vi "FIFOScreenBurst.vi"() -> ()   [LabVIEW 2009]
uses:
  <vilib>/Utility/file.llb/Write To Spreadsheet File (DBL).vi
  <vilib>/Analysis/NI_AALBase.lvlib
  <vilib>/Analysis/NI_AALPro.lvlib
panel:
  in  "get background":bool
  in  "areas and ratio":cluster{dbl, dbl, dbl}
  in  "ratio histogram":dbl[](array[numeric]) format="%0.2f"
  in  "Case Constant\n(See Context Help) 2":bool=TRUE
  in  "Case Constant\n(See Context Help)":bool
  out "MCS":T1(graph)
  out "Lifetime bins":i32=32768
  out "HH":bool=TRUE
  in  "Export times":bool
  in  "Corellate!":bool
  in  "SPC Format":u16(ring)=3 items=["SPC 630 - 32 bit", "SPC 630 - 48 bit", "SPC 830 - 32 bit", "HydraHarp"]
  out "F2 output path":path
  out "channels":u8[](array[numeric])
  out "element":u32
  in  "Acceptor":u8=3
  in  "Transmitter 2":u8=7
  in  "Donor":u8=1
  in  "Transmitter 1":u8=6
  out "T 2":u32
  in  "Correlation":bool
  in  "File Number":u32(slide) max=17 scale=-1.1..17.0
  in  "MCS Export Path (ASCII-File)":path
  out "Busy":bool
  out "donor":i32
  out "T1":i32
  out "all photons":u32
  out "invalid":u32
  out "gaps":u32
  in  "file path":path=path "D:/data/setup test/sim.fifo"
  in  "binning / s":dbl=0.01 format="%.6f"
  out "Save F2":dbl[][](array[numeric]) format="%.2f"
  in  "Export MCS":bool
  in  "Tab Control":T2(tab)=enum."autcorrelation"
  in  "Export Traces":bool
  in  "Trace Export Path (ASCII-File)":path
  in  "shift (photons)":u32=1000
  out "traces":cluster{"SlideTime":dbl[], dbl[]}[](graph)
  out "traces":cluster{dbl, "binning":dbl, "MLE trace":dbl[]}[](graph)
  in  "binning type":u16(ring) items=["seconds", "photons"]
  in  "binning":dbl=0.002 format="%.6f"
  out "sum":u32
  in  "Export Coincidence":bool
  in  "Coincidence Export Path (ASCII-File)":path
  out "coincidence ratio":dbl format="%.2f"
  in  "lateral peaks":u32=6 min=2 max=10 step=2
  in  "center peak (µs)":dbl=1.0 format="%.2f"
  in  "histogram lenght (µs)":dbl=10.0 format="%.2f"
  out "coincidence histogram":T3(graph)
  in  "delay channel 1":bool=TRUE
  in  "TAC range (ns)":dbl=50.0
  in  "export path":path
  in  "export lifetime":bool
  in  "Export Decay":bool
  in  "export decay path":path
  out "lifetime (ns)":dbl[][](array[numeric]) format="%.2f"
  in  "rebinning":u16=1 min=1 max=4096 step=1
  in  "HH Binning / TAC Gain":u16=1
  out "lifetime histogram":T4(graph)
  in  "ch1 (0=sum)":i32
  in  "ch2":i32=1
  in  "ch3":i32=2
  out "selected photons ch3":u32
  out "max value":dbl
  in  "only selected region?":bool
  in  "Pfad":path
  in  "biExp fit":bool
  out "S+B (Hz)":i32
  in  "B":dbl=500.0 format="%.2f"
  in  "skip":i32
  out "F2":dbl
  in  "cross ch2":i32=1
  in  "auto/crossch1":i32
  in  "none/auto/cross":u8
  out "Autocorrelation":cluster{dbl[], "Best Fit":dbl[]}[](graph)
  in  "FCS-Export-Path":path=path "D:/0.001_2000ns_fcs.dat"
  out "diffusion-triplett-model":string="1/N*(1+(r/1-r)*exp(-x*t1))/(1+x/t2)*(1+x/(4*t2))^(-1/2)+o"
  out "Parameters 3":string[](array[string])=["o", "t1", "t2", "N", "r"]
  in  "Initial Guess Coefficient":dbl[](array[numeric])=[0.0, 0.01, 0.18, 0.03, 0.2] format="%.2e"
  out "Parameters 2":string[](array[string])=["o", "t1", "t2", "N", "r"]
  out "Best Fit Coefficient":dbl[][](array[numeric]) format="%.2e"
  in  "freeform":T5={"model"="((1/b)*(1+(a/(1-a))*exp(-x/t1))/(1+x/t2)*(1+x/(4*t2))^(-1/2))+o", "Parameters"=["o", "t1", "t2", "b", "a"], "x"="x"}
  in  "Fit-Type":u8
  out "on2":cluster{"Axis":dbl[], "Histogram":i32[]}(graph)
  out "ChannelsHist":cluster{"Axis":dbl[], "Histogram":i32[]}(graph)
  out "Avg off":dbl format="%.2f"
  out "Avg On":dbl format="%.2f"
  in  "Int-Threshold 2":sgl format="%.2f"
  in  "Int-Threshold":sgl=15.0 format="%.2f"
  out "Offs 0":cluster{"Axis":dbl[], "Histogram":i32[]}(graph)
  out "On plot1":cluster{"Axis":dbl[], "Histogram":i32[]}(graph)
  out "Int Histogram":cluster{"Axis":dbl[], "Histogram":i32[]}(graph)
  out "off":dbl[](array[numeric]) format="%.2f"
  out "on":dbl[](array[numeric]) format="%.2f"
  in  "min bin time (ns)":u32=1000
  in  "Export Correlation":bool
  out "results":T6
  out "Deviation":cluster{dbl[], "Best Fit":dbl[]}[](graph)
  out "Mean Intensity/\nbackground":dbl
  in  "automatic threshold":bool
  out "Statistik F2":dbl[](array[numeric])=[0.0, 0.06084751773049646, 1269.0, 0.47169755424752874, 11.13572770347884, 1.44, 1.0499999999999998, 0.035, 2.525] format="%.2f"
  out "Fn-Values":cluster{dbl, "Value":dbl, dbl[]}[](graph)
  in  "bin / s":dbl=0.5 format="%.6f"
  in  "Export F2":bool
  out "FRET histogram":cluster{"Axis":dbl[], "Histogram":i32[]}[](graph)
  in  "F2-Value Export Path":path=path "D:/Messungen/040901_VHA-Rh110_VHA-Atto590_AMP-PNP/name_1000mus_55bins.dat"
  out "# bursts":i32
  in  "# bins":i32=55
  out "Summe":cluster{"Axis":dbl[], "Histogram":i32[]}(graph)
  in  "% overtalk D-T2":u8
  in  "% overtalk D-A":u8
  in  "% overtalk D-T1":u8
  in  "* w0":u8
  out "mean, std.dev":dbl[](array[numeric])=[0.0, 0.0, -0.3793442467648379, 0.0] format="%.2f"
  in  "Parameters":T7={"PeakThreshold"=30, "RecognitionThs"=25, "SeparationLimit"=0.7} {"SeparationLimit" format="%.2f"}
  in  "Burst recognition":bool=TRUE
  in  "Save ASCII":bool
  in  "add previous":bool
  in  "Open":bool
  in  "Save":bool
  out "# off times":i32
  out "# on times":i32
  out "off time histogram":T8(graph)
  in  "intervals":i32=3
  out "on count histogram":T8(graph)
  out "StdDev":dbl format="%0.2f"
  out "off time (s)":dbl
  out "StdDev":dbl format="%_4f"
  out "off times (s)":dbl[](array[numeric]) format="%.4f"
  out "on counts":i32[](array[numeric])
  out "on time photons":dbl
  in  "channel":i32
  in  "start":bool
  in  "Export area histogram":bool
  in  "Clear histogram":bool
  in  "Add ratio":bool
  out "Histogram Graph":cluster{"X":dbl[], "Histogram":dbl[]}[](graph)
  out "ratio peak areas\nFRET high/FRET low":dbl
  in  "fitting?":bool
  out "ratio histogram":T8(graph)
  out "area low FRET":dbl
  out "area high FRET":dbl
  out "sum low":dbl
  out "sum high":dbl
  # "FifFo Screen Burst\nFour Channel extension\nv0.17"
  # "0: none\n1: diffusion\n2: freeform\n3: exponentiell"
  # "Donor"
  # "Transmitter1"
  # "Transmitter2"
  # "r is amplitude fraction of triplet"
  # "Acceptor"
  # "in ms"
  # "Spot"
  # "burst/s"
  # "bursts"
  # "mean burstwidth /ms"
  # "mean Int"
  # "rec. Thres"
  # "x"
  # "µ"
  # "2*s"
  # "calculates E= acceptor/(acceptor+donor) and fits two gaussian"
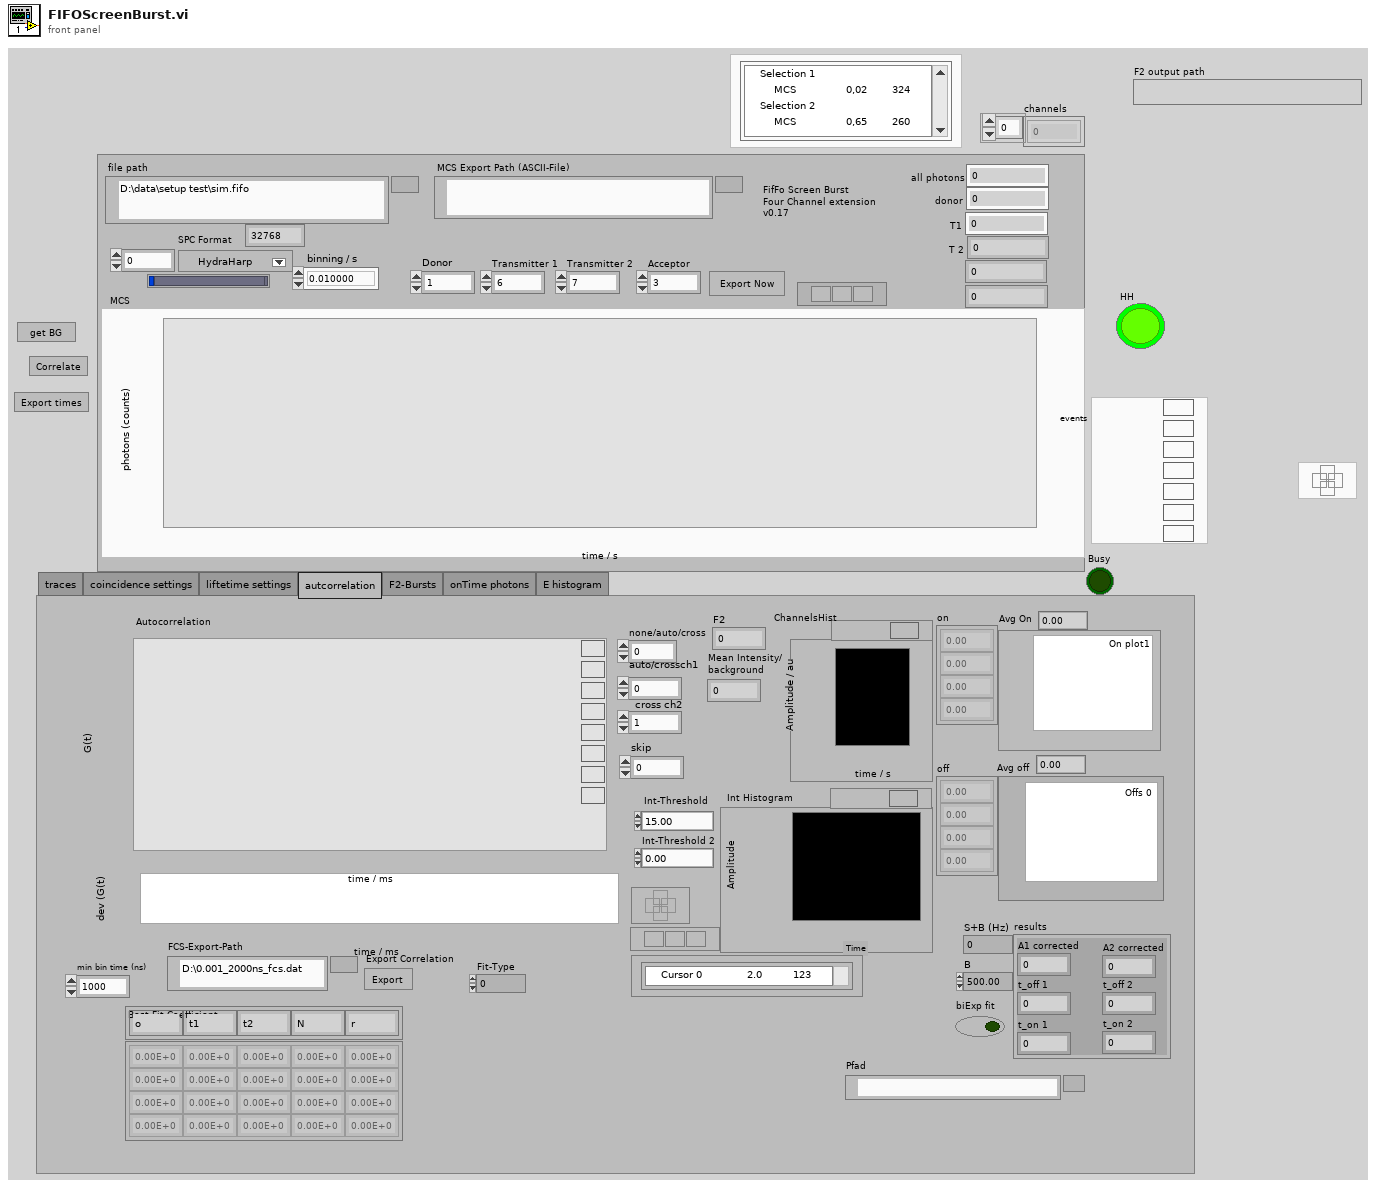
[diagram p1: front panel]
types:
  T1 = cluster{"binning (s)":dbl, "binning (s)":dbl, "Histogram: h(x)":u32[]}[]
  T2 = enum32{"traces", "coincidence settings", "liftetime settings", "autcorrelation", "F2-Bursts", "onTime photons", "E histogram"}
  T3 = cluster{"Origin (ns)":dbl, "Offset (ns)":dbl, u32[]}
  T4 = cluster{dbl, "channel width (ns)":dbl, "channel 1":u32[]}[]
  T5 = cluster{"model":string, "Parameters":string[], "x":string}
  T6 = cluster{"A1 corrected":dbl, "t_off 1":dbl, "t_on 1":dbl, "A2 corrected":dbl, "t_off 2":dbl, "t_on 2":dbl}
  T7 = cluster{"PeakThreshold":u32, "RecognitionThs":u32, "SeparationLimit":sgl}
  T8 = cluster{"X Values":dbl[], "Histogram: h(x)":i32[]}
  T9 = enum16{"open", "open or create", "create or replace", "create", "open (read only)"}
  T10 = cluster{dbl, "binning":dbl, "center peak trace":dbl[]}[]
  T11 = cluster{"SlideTime":dbl[], "SlideCenterPeak":dbl[]}[]
  T12 = cluster{"origin (ns)":dbl, "offset (ns)":dbl, "histogram":u32[]}
  T13 = typedef "Settings.ctl" = cluster{"threshold":cluster{"max":u32, "min":u32}, "RGB or false color":bool, "16bit":bool, "log/lin axis":u16, "spotsize button":bool, "Pixelsize":u16, "autoscale x":bool, "autoscale y":bool, "correlation":bool, "ADC-Resolution":i32, "F2-lifetime":cluster{"display tau":bool, "display F2":bool, "Palette Number lifetime":enum32{"Gray", "Binary", "Gradient", "Rainbow", "Temperature"}, "Palette Number F2":enum32{"Gray", "Binary", "Gradient", "Rainbow", "Temperature"}, "max tau-Value":dbl, "min tau-Value":dbl, "max F2-Value":dbl, "min F2-Value":dbl}, "TAC-Window 1":u16, "TAC-Window 2":u16, "false color palette":cluster{"1":u32, "2":u32, "3":u32, "4":u32, "5":u32, "6":u32, "7":u32, "8":u32, "8 2":u32, "8 3":u32, "8 4":u32, "8 5":u32}, "rebinning":dbl}
  T14 = cluster{"sum":u32[], "channel 0":u32[], "channel 1":u32[], "channel width (ns)":dbl}
  T15 = typedef "LVCursorListTypeDef.ctl" = cluster{"Name":string, "Color":u32, "Style":u8, "Point Style":u8, "Name Visible":bool, "Allow Drag":bool, "Cursor Mode":u32, "Plot":i32, "Index":i32, "Position":cluster{"X":dbl, "Y":dbl}, "X Scale":u32, "Y Scale":u32, "Watch Plots":i32[], "Watch All Plots":bool, "Plot Area":i32, "Label Offset":cluster{"X":dbl, "Y":dbl}}[]
  T16 = cluster{"router channels":u8[], "macro times":dbl[], "micro times":u16[], "invalid times":u32[], "gap times":u32[]}
  T17 = cluster{"Name":string, "Color":u32, "Style":u8, "Point Style":u8, "Name Visible":bool, "Allow Drag":bool, "Cursor Mode":u32, "Plot":i32, "Index":i32, "Position":cluster{"X":dbl, "Y":dbl}, "X Scale":u32, "Y Scale":u32, "Watch Plots":i32[], "Watch All Plots":bool, "Plot Area":i32, "Label Offset":cluster{"X":dbl, "Y":dbl}}
  T18 = cluster{"binning (s)":dbl, "binning (s)":dbl, "Histogram: h(x)":u32[]}
  T19 = cluster{"router channels":u8[], "macro times(50ns steps)":u32[], "micro times":u16[], "invalid times":u32[], "gap times":u32[]}
  T20 = cluster{"router channels":u8[], "macro times":u32[], "micro times":u16[], "invalid times":u32[], "gap times":u32[]}
  T21 = cluster{"binning (s)":dbl, "binning (s)":dbl, "Histogram: h(x)":i32[]}
  T22 = cluster{"offset":dbl, "binning (s)":dbl, "MCS":u32[]}
  T23 = cluster{"binning (s)":dbl, "binning (s)":dbl, "MCS":u32[]}[]
  T24 = cluster{dbl, "binning":dbl, "coincidence trace":dbl[]}
  T25 = cluster{dbl, "binning":dbl, "center peak trace":u32[]}
  T26 = cluster{dbl, "binning":dbl, "coincidence trace":dbl[]}[]
  T27 = cluster{"SlideTime":dbl[], "SlideLifetime":dbl[]}
  T28 = cluster{"SlideTime":dbl[], "SlideCoincidence":dbl[]}
  T29 = cluster{"SlideTime":dbl[], "SlideCenterPeak":u32[]}
  T30 = cluster{"SlideTime":dbl[], "SlideCoincidence":dbl[]}[]
  T31 = cluster{dbl, "channel width (ns)":dbl, "sum":u32[]}
  T32 = cluster{dbl, "channel width (ns)":dbl, "channel 0":u32[]}
  T33 = cluster{dbl, "channel width (ns)":dbl, "channel 1":u32[]}
  T34 = cluster{"PeakThreshold":u32, "RecognitionThreshold":u32, "SeparationLimit":sgl}
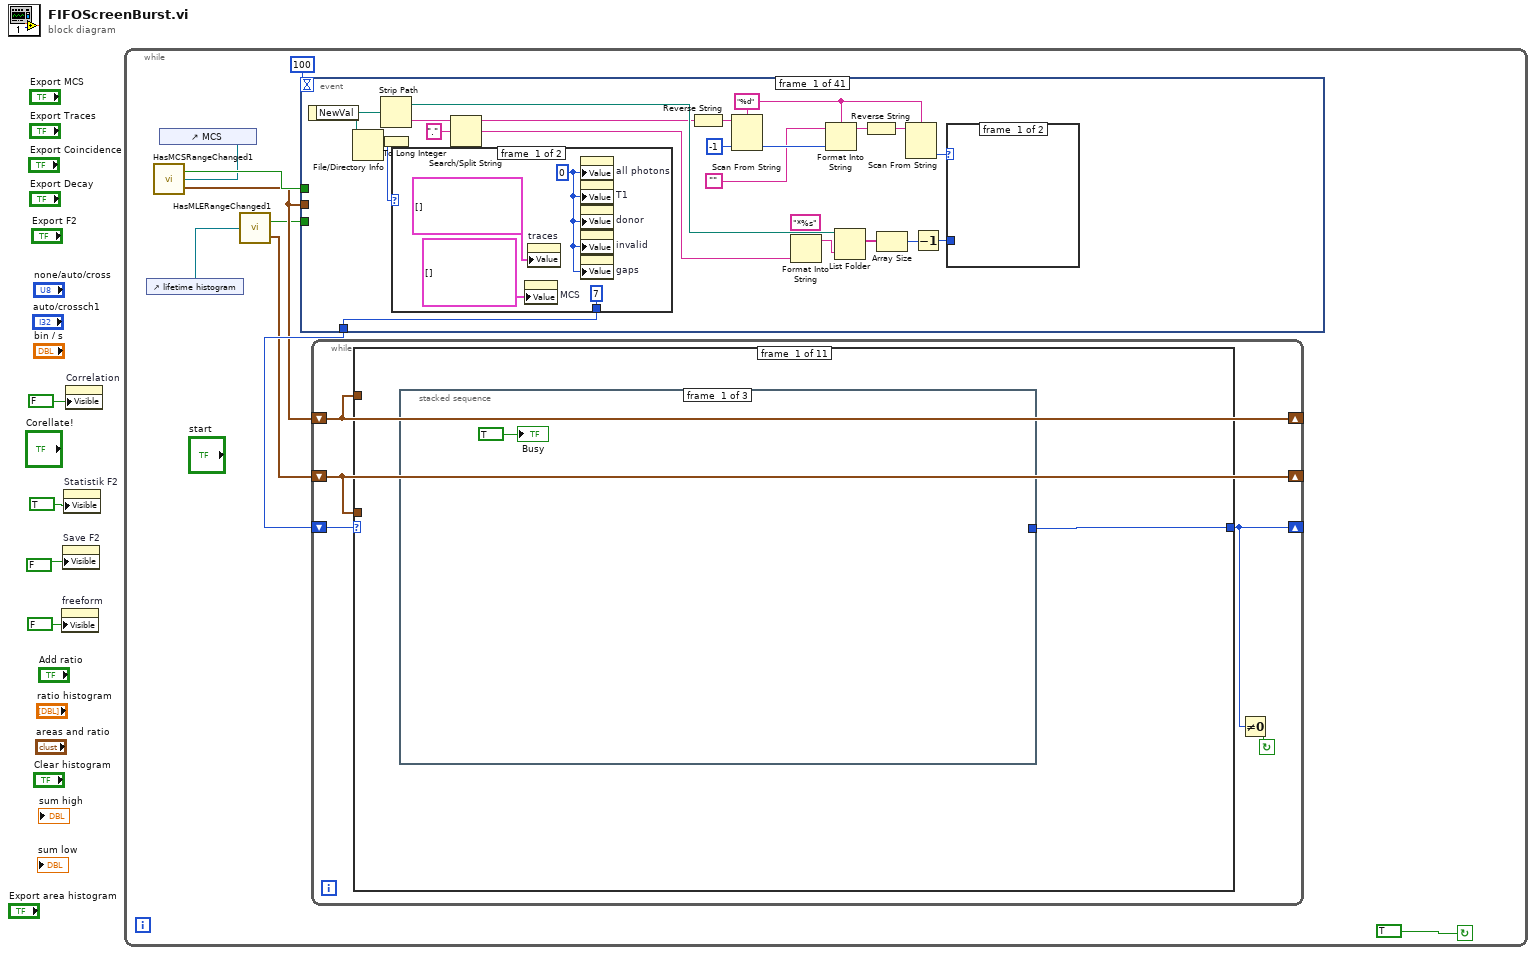
[diagram p0: block diagram]
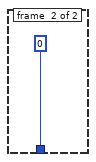
[diagram p2: hidden frame]
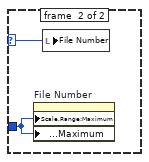
[diagram p3: hidden frame]
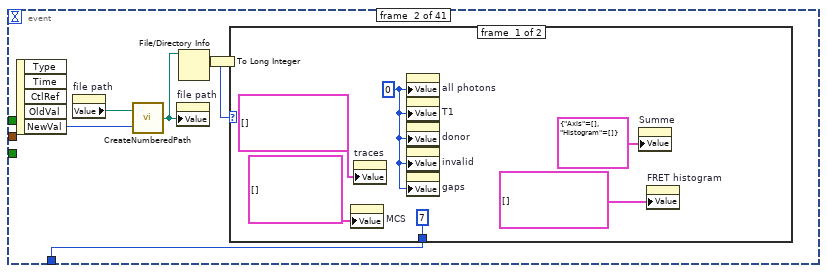
[diagram p4: hidden frame]
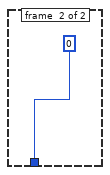
[diagram p5: hidden frame]
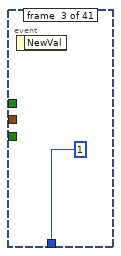
[diagram p6: hidden frame]
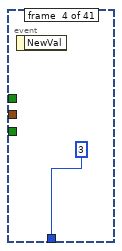
[diagram p7: hidden frame]
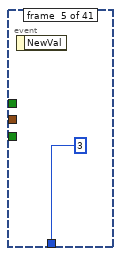
[diagram p8: hidden frame]
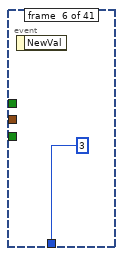
[diagram p9: hidden frame]
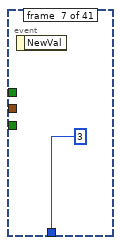
[diagram p10: hidden frame]
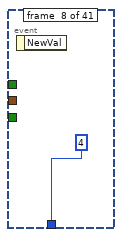
[diagram p11: hidden frame]
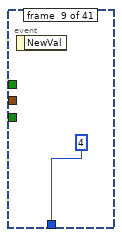
[diagram p12: hidden frame]
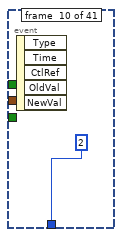
[diagram p13: hidden frame]
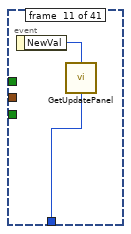
[diagram p14: hidden frame]
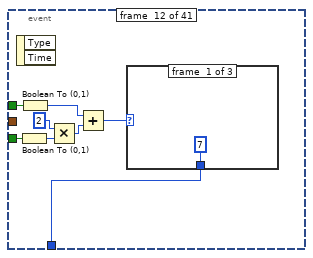
[diagram p15: hidden frame]
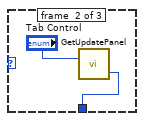
[diagram p16: hidden frame]
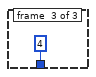
[diagram p17: hidden frame]
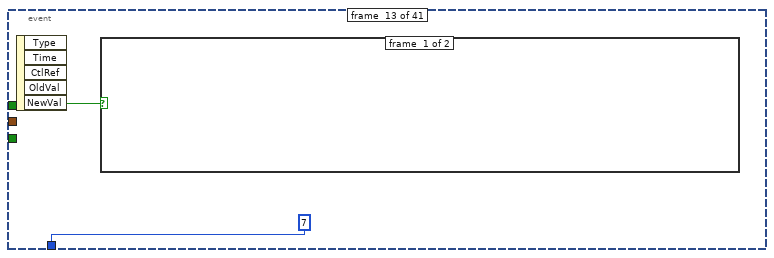
[diagram p18: hidden frame]
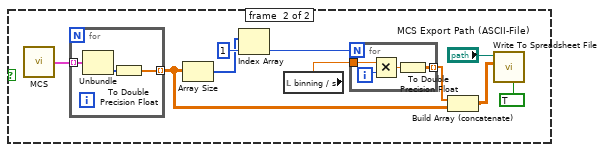
[diagram p19: hidden frame]
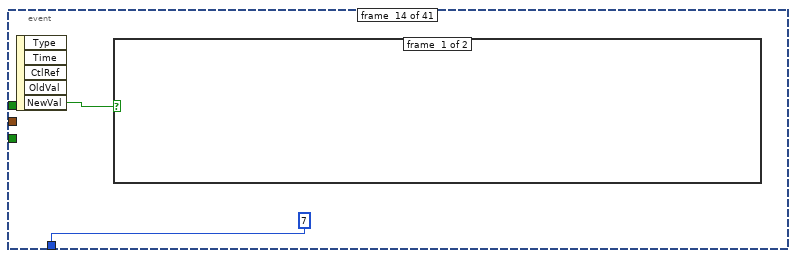
[diagram p20: hidden frame]
diagram:
  n1 = property on="freeform" class="Cluster (strict)"("Visible"=FALSE) -> ()  [unwired: 2 in, 2 out]
  n2 = property on="Save F2" class="Array (strict)"("Visible"=FALSE) -> ()  [unwired: 2 in, 2 out]
  n3 = property on="Statistik F2" class="Array (strict)"("Visible"=TRUE) -> ()  [unwired: 2 in, 2 out]
  n4 = property on="Correlation" class="Boolean"("Visible"=FALSE) -> ()  [unwired: 2 in, 2 out]
  n5 = while {
    stop <- TRUE continue-if-true
    n6 = control-ref of="lifetime histogram"() -> (w6:refnum<vi>)
    n7 = control-ref of="MCS"() -> (w7:refnum<vi>)
    n8 = call "HasMCSRangeChanged1.vi"("WFGraph Refnum"=w7) -> ("Selection Changed"=w11:bool, "output range"=w10:cluster{"x0":dbl, "x1":dbl})
    n9 = call "HasMLERangeChanged1.vi"("WFGraph Refnum"=w6) -> ("Selection Changed"=w9:bool, "output range"=w8:cluster{"x0":dbl, "x1":dbl})
    n10 = event shown="[31] \"get background\": Value Change" {
      selector: _ -> [_ _ _ _ _ _ _ _ _ _ _ _ _ _ _ _ _ _ _ _ _ _ _ _ _ _ _ _ _ _ _ _ _ _ _ _ _ _ _ _ _]
      dyn-events: _ -> [_ _ _ _ _ _ _ _ _ _ _ _ _ _ _ _ _ _ _ _ _ _ _ _ _ _ _ _ _ _ _ _ _ _ _ _ _ _ _ _ _]
      timeout: 100 -> [_ _ _ _ _ _ _ _ _ _ _ _ _ _ _ _ _ _ _ _ _ _ _ _ _ _ _ _ _ _ _ _ _ _ _ _ _ _ _ _ _]
      tunnel: [w35 w45 1 3 3 3 3 u32 4 ("Numeric") u32 4 ("Numeric") u32 2 ("Numeric") w64 w73 u32 7 ("Numeric") u32 7 ("Numeric") u32 7 ("Numeric") u32 7 ("Numeric") _ u32 7 ("Numeric") u32 7 ("Numeric") u32 0 ("Numeric") u32 6 ("Numeric") u32 1 ("Numeric") u32 1 ("Numeric") u32 1 ("Numeric") u32 1 ("Numeric") u32 7 ("Numeric") u32 6 ("Numeric") u32 6 ("Numeric") u32 6 ("Numeric") u32 6 ("Numeric") u32 5 ("Numeric") _ u32 6 ("Numeric") w293 u32 9 ("Numeric") u32 7 ("Numeric") u32 9 ("Numeric") u32 7 ("Numeric") _ _ _] -> w12
      tunnel: w11 -> [_ _ _ _ _ _ _ _ _ _ _ w72 _ _ _ _ _ _ _ _ _ _ _ _ _ _ _ _ _ _ _ _ _ _ _ _ _ _ _ _ _]
      tunnel: w9 -> [_ _ _ _ _ _ _ _ _ _ _ w71 _ _ _ _ _ _ _ _ _ _ _ _ _ _ _ _ _ _ _ _ _ _ _ _ _ _ _ _ _]
      tunnel: w10 -> [_ _ _ _ _ _ _ _ _ _ _ _ _ _ _ _ _ _ _ w213 _ _ _ _ _ _ _ _ _ _ _ _ _ _ _ _ _ _ _ _ _]
      event #0 {
        w15 = "%d" ("format string")
        n11 = event-data() -> ("NewVal"=w18:path)  [unwired: 1 in]
        n12 = File/Directory Info(path=w18) -> (size=w14:i64)  [unwired: 1 in, 6 out]
        n13 = Strip Path(path=w18) -> (stripped path=w32:path, name=w33:string)
        n14 = To Long Integer(number=w14) -> (32bit integer=w17:i32)
        n15 = case shown="0" w17 {
          tunnel: [7 0] -> w35
          frame #0 {
            w38 = u32 0 ("photons")
            n16 = property on="MCS" class="WFGraph (strict)"("Value"=T1 [] ("MCS")) -> ()  [unwired: 2 in, 2 out]
            n17 = property on="traces" class="XYGraph (strict)"("Value"=cluster{"SlideTime":dbl[], dbl[]}[] [] ("traces")) -> ()  [unwired: 2 in, 2 out]
            n18 = property on="all photons" class="Digital (strict)"("Value"=w38) -> ()  [unwired: 2 in, 2 out]
            n19 = property on="T1" class="DigNum (strict)"("Value"=w38) -> ()  [unwired: 2 in, 2 out]
            n20 = property on="donor" class="DigNum (strict)"("Value"=w38) -> ()  [unwired: 2 in, 2 out]
            n21 = property on="invalid" class="DigNum (strict)"("Value"=w38) -> ()  [unwired: 2 in, 2 out]
            n22 = property on="gaps" class="DigNum (strict)"("Value"=w38) -> ()  [unwired: 2 in, 2 out]
          }
          frame #1 {
          }
        }
        n23 = Search/Split String(string=w33, search string/char (-)=".") -> (substring before match=w25:string, match + rest of string=w30:string)  [unwired: 1 in, 1 out]
        n24 = Reverse String(1:w25) -> (0:w27:string)
        n25 = Scan From String(format string=w15, input string=w27, default 1=-1 ("default value 1")) -> (output 1=w22:i32)  [unwired: 2 in, 3 out]
        n26 = Format Into String(format string="*%s", w30) -> (resulting string=w29:string)  [unwired: 2 in, 1 out]
        n27 = Format Into String(format string=w15, initial string="", w22) -> (resulting string=w21:string)  [unwired: 1 in, 1 out]
        n28 = List Folder(path=w32, pattern=w29) -> (filenames=w28:string[])  [unwired: 2 in, 3 out]
        n29 = Reverse String(1:w21) -> (0:w19:string)
        n30 = Array Size(array=w28) -> (size(s)=w24:i32)
        n31 = Scan From String(format string=w15, input string=w19) -> (output 1=w20:i32)  [unwired: 3 in, 3 out]
        n32 = Decrement(x=w24) -> (x-1=w23:i32)
        n33 = case shown="0, Default" w20 {
          selector: w20 -> [_ w41]
          tunnel: w23 -> [_ w42]
          frame #0 {
          }
          frame #1 {
            n34 = property on="File Number" class="Slide (strict)"("Scale.Range:Maximum"=w42, "Data Entry Limits:Maximum"=w42) -> ()  [unwired: 2 in, 2 out]
            n35 = local write "File Number"(w41) -> ()
          }
        }
      }
      event #1 {
        n36 = event-data() -> ("NewVal"=w48:u32)  [unwired: 1 in, 4 out]
        n37 = property on="file path" class="Path"() -> ("Value"=w47:path)  [unwired: 2 in, 2 out]
        n38 = call "CreateNumberedPath.vi"("File Number"=w48, "file path"=w47) -> ("Path"=w46:path)
        n39 = property on="file path" class="Path"("Value"=w46) -> ()  [unwired: 2 in, 2 out]
        n40 = File/Directory Info(path=w46) -> (size=w43:i64)  [unwired: 1 in, 6 out]
        n41 = To Long Integer(number=w43) -> (32bit integer=w44:i32)
        n42 = case shown="0" w44 {
          tunnel: [7 0] -> w45
          frame #0 {
            w53 = u32 0 ("photons")
            n43 = property on="MCS" class="WFGraph (strict)"("Value"=T1 [] ("MCS")) -> ()  [unwired: 2 in, 2 out]
            n44 = property on="traces" class="XYGraph (strict)"("Value"=cluster{"SlideTime":dbl[], dbl[]}[] [] ("traces")) -> ()  [unwired: 2 in, 2 out]
            n45 = property on="all photons" class="DigNum (strict)"("Value"=w53) -> ()  [unwired: 2 in, 2 out]
            n46 = property on="T1" class="DigNum (strict)"("Value"=w53) -> ()  [unwired: 2 in, 2 out]
            n47 = property on="donor" class="DigNum (strict)"("Value"=w53) -> ()  [unwired: 2 in, 2 out]
            n48 = property on="invalid" class="DigNum (strict)"("Value"=w53) -> ()  [unwired: 2 in, 2 out]
            n49 = property on="gaps" class="DigNum (strict)"("Value"=w53) -> ()  [unwired: 2 in, 2 out]
            n50 = property on="Summe" class="XYGraph (strict)"("Value"=cluster{"Axis":dbl[], "Histogram":i32[]} {"Axis"=[], "Histogram"=[]} ("Summe")) -> ()  [unwired: 2 in, 2 out]
            n51 = property on="FRET histogram" class="XYGraph (strict)"("Value"=cluster{"Axis":dbl[], "Histogram":i32[]}[] [] ("FRET histogram")) -> ()  [unwired: 2 in, 2 out]
          }
          frame #1 {
          }
        }
      }
      event #2 {
        n52 = event-data() -> ()  [unwired: 1 in, 1 out]
      }
      event #3 {
        n53 = event-data() -> ()  [unwired: 1 in, 1 out]
      }
      event #4 {
        n54 = event-data() -> ()  [unwired: 1 in, 1 out]
      }
      event #5 {
        n55 = event-data() -> ()  [unwired: 1 in, 1 out]
      }
      event #6 {
        n56 = event-data() -> ()  [unwired: 1 in, 1 out]
      }
      event #7 {
        n57 = event-data() -> ()  [unwired: 1 in, 1 out]
      }
      event #8 {
        n58 = event-data() -> ()  [unwired: 1 in, 1 out]
      }
      event #9 {
        n59 = event-data() -> ()  [unwired: 1 in, 5 out]
      }
      event #10 {
        n60 = event-data() -> ("NewVal"=w65:T2)  [unwired: 1 in]
        n61 = call "GetUpdatePanel.vi"("Tab Control"=w65) -> ("Numeric"=w64:u32)
      }
      event #11 {
        n62 = event-data() -> ()  [unwired: 1 in, 2 out]
        n63 = Boolean To (0,1)(Boolean=w71) -> (0, 1=w70:i16)
        n64 = Boolean To (0,1)(Boolean=w72) -> (0, 1=w67:i16)
        n65 = Multiply(x=i16 2, y=w70) -> (x*y=w68:i16)
        n66 = Add(x=w67, y=w68) -> (x+y=w66:i16)
        n67 = case shown="1" w66 {
          tunnel: [u32 7 ("Numeric") w75 u32 4 ("Numeric")] -> w73
          frame #0 {
          }
          frame #1 {
            n68 = call "GetUpdatePanel.vi"("Tab Control"="Tab Control") -> ("Numeric"=w75:u32)
          }
          frame #2 {
          }
        }
      }
      event #12 {
        n69 = event-data() -> ("NewVal"=w79:bool)  [unwired: 1 in, 4 out]
        n70 = case shown="True" w79 {
          frame #0 {
          }
          frame #1 {
            n71 = call "MCS.vi"() -> ("MCS output"=w89:T1)  [unwired: 2 in]
            n72 = for {
              tunnel: w89 -> [w96] mode=indexing
              tunnel: [w94] -> w83 mode=indexing
              n73 = Unbundle(w96) -> ("Histogram: h(x)"=w95:u32[])  [unwired: 2 out]
              n74 = To Double Precision Float(number=w95) -> (double precision float=w94:dbl[])
            }
            n75 = Array Size(array=w83) -> (size(s)=w80:i32[])
            n76 = Index Array(array=w80, index=1) -> (element=w82:i32)
            n77 = local read "binning / s"() -> (w85:dbl)
            n78 = for {
              N: w82 -> [_]
              tunnel: w85 -> [w93]
              tunnel: [w90] -> w84 mode=indexing
              i -> [w92]
              n79 = Multiply(x=w93, y=w92) -> (x*y=w91:dbl)
              n80 = To Double Precision Float(number=w91) -> (double precision float=w90:dbl)
            }
            n81 = Build Array (concatenate)(w84, w83) -> (w88:dbl[][])
            n82 = call-poly <vilib>:"Write To Spreadsheet File.vi"("transpose? (no:F)"=TRUE, "2D data"=w88, "file path (dialog if empty)"="MCS Export Path (ASCII-File)") -> ()  [unwired: 5 in, 1 out]
          }
        }
      }
      event #13 {
        n83 = event-data() -> ("NewVal"=w98:bool)  [unwired: 1 in, 4 out]
        n84 = case shown="True" w98 {
          frame #0 {
          }
          frame #1 {
            n85 = local read "binning type"() -> (w100:u16)
            n86 = case shown="0, Default" w100 {
              tunnel: "Trace Export Path (ASCII-File)" -> [w102 w116]
              frame #0 {
                n87 = call "BinningTraces.vi"() -> ("binned traces out"=w110:T10)  [unwired: 2 in]
                n88 = for {
                  tunnel: w110 -> [w115] mode=indexing
                  tunnel: [w114] -> w104 mode=indexing
                  n89 = Unbundle(w115) -> ("center peak trace"=w114:dbl[])  [unwired: 2 out]
                }
                n90 = Array Size(array=w104) -> (size(s)=w109:i32[])
                n91 = Index Array(array=w109, index=1) -> (element=w107:i32)
                n92 = local read "binning"() -> (w106:dbl)
                n93 = for {
                  N: w107 -> [_]
                  tunnel: w106 -> [w113]
                  tunnel: [w111] -> w105 mode=indexing
                  i -> [w112]
                  n94 = Multiply(x=w113, y=w112) -> (x*y=w111:dbl)
                }
                n95 = Build Array (concatenate)(w105, w104) -> (w103:dbl[][])
                n96 = call-poly <vilib>:"Write To Spreadsheet File.vi"("transpose? (no:F)"=TRUE, "2D data"=w103, "file path (dialog if empty)"=w102) -> ()  [unwired: 5 in, 1 out]
              }
              frame #1 {
                n97 = call "SlidingTraces.vi"() -> ("sliding traces out"=w121:T11)  [unwired: 2 in]
                n98 = for {
                  tunnel: w121 -> [w124] mode=indexing
                  tunnel: [w123] -> w119 mode=indexing
                  tunnel: [w122] -> w120
                  n99 = Unbundle(w124) -> ("SlideTime"=w122:dbl[], "SlideCenterPeak"=w123:dbl[])
                }
                n100 = Build Array (concatenate)(w120, w119) -> (w118:dbl[][])
                n101 = call-poly <vilib>:"Write To Spreadsheet File.vi"("transpose? (no:F)"=TRUE, "2D data"=w118, "file path (dialog if empty)"=w116) -> ()  [unwired: 5 in, 1 out]
              }
            }
          }
        }
      }
      event #14 {
        n102 = event-data() -> ("NewVal"=w125:bool)  [unwired: 1 in, 4 out]
        n103 = case shown="True" w125 {
          frame #0 {
          }
          frame #1 {
            n104 = call "CoincidenceHistogram.vi"() -> ("coincidence histogram out"=w135:T12)  [unwired: 2 in]
            n105 = Unbundle(w135) -> ("offset (ns)"=w133:dbl, "histogram"=w132:u32[])  [unwired: 1 out]
            n106 = Array Size(array=w132) -> (size(s)=w134:i32)
            n107 = for {
              N: w134 -> [_]
              tunnel: w133 -> [w138]
              tunnel: [w136] -> w131 mode=indexing
              i -> [w137]
              n108 = Multiply(x=w138, y=w137) -> (x*y=w136:dbl)
            }
            n109 = To Double Precision Float(number=w132) -> (double precision float=w130:dbl[])
            n110 = Build Array(w131, w130) -> (w129:dbl[][])
            n111 = call-poly <vilib>:"Write To Spreadsheet File.vi"("transpose? (no:F)"=TRUE, "2D data"=w129, "file path (dialog if empty)"="Coincidence Export Path (ASCII-File)") -> ()  [unwired: 5 in, 1 out]
          }
        }
      }
      event #15 {
        n112 = event-data() -> ("NewVal"=w140:bool)  [unwired: 1 in, 4 out]
        n113 = case shown="True" w140 {
          frame #0 {
          }
          frame #1 {
            n114 = flat-sequence {
              frame #0 {
                # "rebinning already accounted for in channel width\nStd Settings needed for export fluofit (time in x rebinning)"
                n115 = call "StandardSettings.vi"("Enum"=enum16{"Load", "get", "Save", "set"}."get") -> ("StandardSettings"=w143:T13)  [unwired: 4 in]
                n116 = Bundle By Name(cluster=w143, "rebinning"=1.0) -> (w142:T13)
                n117 = call "StandardSettings.vi"("StandardSettings"=w142, "Enum"=enum16{"Load", "get", "Save", "set"}."set") -> ()  [unwired: 3 in, 1 out]
              }
              frame #1 {
                n118 = call "LifetimeHistograms.vi"() -> ("output lifetime histograms"=w165:T14)  [unwired: 2 in]
                n119 = Unbundle(w165) -> ("sum"=w162:u32[], "channel 0"=w161:u32[], "channel 1"=w160:u32[], "channel width (ns)"=w164:dbl)
                n120 = Array Size(array=w162) -> (size(s)=w163:i32)
                n121 = property on="lifetime histogram" class="WFGraph (strict)"() -> ("CrsrList"=w148:T15)  [unwired: 2 in, 2 out]
                n122 = To Double Precision Float(number=w162) -> (double precision float=w158:dbl[])
                n123 = for {
                  N: w163 -> [_]
                  tunnel: w164 -> [w167]
                  tunnel: [w166] -> w159 mode=indexing
                  i -> [w168]
                  n124 = Multiply(x=w167, y=w168) -> (x*y=w166:dbl)
                }
                n125 = To Double Precision Float(number=w161) -> (double precision float=w157:dbl[])
                n126 = To Double Precision Float(number=w160) -> (double precision float=w156:dbl[])
                n127 = call "selectDecayRegion.vi"("Cursor List"=w148, "only selected region?"="only selected region?", "histogram 3"=w156, "histogram 2"=w157, "histogram 1"=w158, "time in"=w159) -> ("histogram 3 out"=w155:dbl[], "histogram2 out"=w154:dbl[], "histogram 1 out"=w153:dbl[], "time out"=w150:dbl[])
                n128 = Array Size(array=w150) -> (size(s)=w149:i32)
                n129 = Build Array(w153, w154, w155) -> (w151:dbl[][])
                n130 = call "ExportFluoFit.vi"("from end?"=FALSE, "time in"=w150, "# of lines"=w149, "lifetimes"=w151, "Lifetime Export Path (ASCII-File)"="export decay path") -> ()  [unwired: 2 in]
              }
            }
          }
        }
      }
      event #16 {
        n131 = event-data() -> ()  [unwired: 1 in, 5 out]
        n132 = case shown="True" "Export Correlation" {
          tunnel: [w175 w189] -> w171
          tunnel: "FCS-Export-Path" -> [w174 w185]
          frame #0 {
            n133 = property on="file path" class="Path"() -> ("Value"=w173:path)  [unwired: 2 in, 2 out]
            n134 = property on="min bin time (ns)" class="Digital (strict)"() -> ("Value"=w172:u32)  [unwired: 2 in, 2 out]
            n135 = call "FCS_Automatic_Filename_sub.vi"("bin / ns"=w172, "FCS save directory"=w174, "file path"=w173) -> ("FCS output path"=w175:path)
          }
          frame #1 {
            n136 = property on="file path" class="Path"() -> ("Value"=w184:path)  [unwired: 2 in, 2 out]
            n137 = property on="min bin time (ns)" class="Digital (strict)"() -> ("Value"=w188:u32)  [unwired: 2 in, 2 out]
            n138 = property on="Fit-Type" class="Digital (strict)"() -> ("Value"=w187:u8)  [unwired: 2 in, 2 out]
            n139 = Add(x=w188, y=w187) -> (x+y=w186:u32)
            n140 = call "FCS_Automatic_Filename_sub.vi"("bin / ns"=w188, "FCS save directory"=w185, "file path"=w184) -> ("FCS output path"=w189:path)
            n141 = call "FCS_Automatic_Filename_sub.vi"("bin / ns"=w186, "FCS save directory"=w185, "file path"=w184) -> ("FCS output path"=w183:path)
            n142 = property on="Autocorrelation" class="XYGraph (strict)"() -> ("Value"=w176:cluster{dbl[], "Best Fit":dbl[]}[])  [unwired: 2 in, 2 out]
            n143 = property on="Best Fit Coefficient" class="Array (strict)"() -> ("Value"=w182:dbl[][])  [unwired: 2 in, 2 out]
            n144 = call "FCScluster2SaveArray_sub.vi"("Autocorrelation"=w176) -> ("FCS-Data"=w181:dbl[][])  [unwired: 2 in]
            n145 = call-poly <vilib>:"Write To Spreadsheet File.vi"("transpose? (no:F)"=FALSE, "append to file? (new file:F)"=TRUE, "2D data"=w182, "file path (dialog if empty)"=w183) -> ()  [unwired: 4 in, 1 out]
            n146 = call-poly <vilib>:"Write To Spreadsheet File.vi"("transpose? (no:F)"=TRUE, "append to file? (new file:F)"=TRUE, "2D data"=w181, "file path (dialog if empty)"=w189) -> ()  [unwired: 4 in, 1 out]
          }
        }
        n147 = property on="FCS-Export-Path" class="Path"("Value"=w171) -> ()  [unwired: 2 in, 2 out]
      }
      event #17 {
        n148 = event-data() -> ()  [unwired: 1 in, 6 out]
        n149 = case shown="True" "Export times" {
          frame #0 {
          }
          frame #1 {
            n150 = property on="results" class="Clust (strict)"() -> ("Value"=w199:T6)  [unwired: 2 in, 2 out]
            n151 = property on="all photons" class="Digital (strikt)"() -> ("Value"=w193:u32)  [unwired: 2 in, 2 out]
            n152 = Unbundle(w199) -> ("t_off 1"=w198:dbl, "t_on 1"=w197:dbl, "t_off 2"=w196:dbl, "t_on 2"=w195:dbl)  [unwired: 2 out]
            n153 = Build Array(w193, w198, w197, w196, w195) -> (w192:dbl[])
            n154 = call-poly <vilib>:"Write To Spreadsheet File.vi"("append to file? (new file:F)"=TRUE, "1D data"=w192, "file path (dialog if empty)"="Pfad") -> ()  [unwired: 5 in, 1 out]
          }
        }
      }
      event #18 {
        n155 = event-data() -> ()  [unwired: 1 in, 6 out]
        n156 = case shown="True" "export lifetime" {
          frame #0 {
          }
          frame #1 {
            n157 = property on="lifetime (ns)" class="Array (strikt)"() -> ("Value"=w208:dbl[][])  [unwired: 2 in, 2 out]
            n158 = Array Subset(array=w208, index (row)=0 ("Index"), length (row)=1 ("Länge"), index (col)=0 ("Index"), length (col)=1 ("Länge")) -> (w203:dbl[][])
            n159 = call-poly <vilib>:"Write To Spreadsheet File.vi"("append to file? (new file:F)"=TRUE, "2D data"=w203, "file path (dialog if empty)"="export path") -> ()  [unwired: 5 in, 1 out]
          }
        }
      }
      event #19 {
        n160 = event-data() -> ()  [unwired: 1 in, 5 out]
        n161 = case shown="True" "Correlation" {
          tunnel: w213 -> [_ w216]
          frame #0 {
          }
          frame #1 {
            n162 = call "MCS.vi"() -> ("MCS output"=w215:T1)  [unwired: 2 in]
            n163 = property on="binning / s" class="Digital (strict)"() -> ("Value"=w214:dbl)  [unwired: 2 in, 2 out]
            n164 = call "Rawdata.vi"() -> ("output rawdata"=w217:T16)  [unwired: 2 in]
            n165 = call "correlation.vi"("selection range"=w216, "binning"=w214, "MCS"=w215, "rawdata"=w217) -> ()
          }
        }
      }
      event #20 {
        n166 = event-data() -> ()  [unwired: 1 in, 5 out]
      }
      event #21 {
        n167 = event-data() -> ()  [unwired: 1 in, 5 out]
        n168 = call "MCS.vi"("MCS input"=T1 [], "set"=TRUE) -> ()  [unwired: 1 out]
      }
      event #22 {
        n169 = event-data() -> ()  [unwired: 1 in, 5 out]
        n170 = call "MCS.vi"("MCS input"=T1 [], "set"=TRUE) -> ()  [unwired: 1 out]
      }
      event #23 {
        n171 = event-data() -> ()  [unwired: 1 in, 5 out]
        n172 = call "MCS.vi"("MCS input"=T1 [], "set"=TRUE) -> ()  [unwired: 1 out]
      }
      event #24 {
        n173 = event-data() -> ()  [unwired: 1 in, 5 out]
        n174 = call "MCS.vi"("MCS input"=T1 [], "set"=TRUE) -> ()  [unwired: 1 out]
      }
      event #25 {
        n175 = event-data() -> ("NewVal"=w232:bool)  [unwired: 1 in, 4 out]
        n176 = local read "Burst recognition"() -> (w231:bool)
        n177 = case shown="True" w231 {
          tunnel: w232 -> [_ w235]
          frame #0 {
          }
          frame #1 {
            n178 = case shown="True" w235 {
              tunnel: [w244 w250] -> w236
              tunnel: "F2-Value Export Path" -> [w243 w247]
              frame #0 {
                n179 = property on="binning / s" class="Digital (strict)"() -> ("Value"=w240:dbl)  [unwired: 2 in, 2 out]
                n180 = property on="# bins" class="Digital (strict)"() -> ("Value"=w237:i32)  [unwired: 2 in, 2 out]
                n181 = Multiply(x=w240, y=u32 1000000) -> (x*y=w242:dbl)
                n182 = property on="file path" class="Path"() -> ("Value"=w238:path)  [unwired: 2 in, 2 out]
                n183 = To Unsigned Long Integer(number=w242) -> (unsigned 32bit integer=w239:u32)
                n184 = call "Automatic_FileName_sub.vi"("#bin-histogram"=w237, "bin / ms"=w239, "F2 save directory"=w243, "file path"=w238) -> ("F2 output path"=w244:path)
              }
              frame #1 {
                n185 = property on="# bins" class="Digital (strict)"() -> ("Value"=w245:i32)  [unwired: 2 in, 2 out]
                n186 = property on="binning / s" class="Digital (strict)"() -> ("Value"=w252:dbl)  [unwired: 2 in, 2 out]
                n187 = property on="file path" class="Path"() -> ("Value"=w246:path)  [unwired: 2 in, 2 out]
                n188 = Multiply(x=w252, y=u32 1000000) -> (x*y=w256:dbl)
                n189 = To Unsigned Long Integer(number=w256) -> (unsigned 32bit integer=w251:u32)
                n190 = Increment(x=w251) -> (x+1=w248:u32)
                n191 = call "Automatic_FileName_sub.vi"("#bin-histogram"=w245, "bin / ms"=w251, "F2 save directory"=w247, "file path"=w246) -> ("F2 output path"=w250:path)
                n192 = call "Automatic_FileName_sub.vi"("#bin-histogram"=w245, "bin / ms"=w248, "F2 save directory"=w247, "file path"=w246) -> ("F2 output path"=w249:path)
                n193 = property on="Statistik F2" class="Array (strict)"() -> ("Value"=w254:dbl[])  [unwired: 2 in, 2 out]
                n194 = property on="Save F2" class="Array (strict)"() -> ("Value"=w253:dbl[][])  [unwired: 2 in, 2 out]
                n195 = call-poly <vilib>:"Write To Spreadsheet File.vi"("transpose? (no:F)"=FALSE, "append to file? (new file:F)"=TRUE, "1D data"=w254, "file path (dialog if empty)"=w249) -> ()  [unwired: 4 in, 1 out]
                n196 = call-poly <vilib>:"Write To Spreadsheet File.vi"("transpose? (no:F)"=TRUE, "append to file? (new file:F)"=TRUE, "2D data"=w253, "file path (dialog if empty)"=w250) -> ()  [unwired: 4 in, 1 out]
              }
            }
            n197 = property on="F2-Value Export Path" class="Path"("Value"=w236) -> ()  [unwired: 2 in, 2 out]
          }
        }
      }
      event #26 {
        n198 = event-data() -> ()  [unwired: 1 in, 5 out]
      }
      event #27 {
        n199 = event-data() -> ()  [unwired: 1 in, 5 out]
      }
      event #28 {
        n200 = event-data() -> ()  [unwired: 1 in, 5 out]
      }
      event #29 {
        n201 = event-data() -> ()  [unwired: 1 in, 5 out]
      }
      event #30 {
        n202 = event-data() -> ()  [unwired: 1 in, 4 out]
      }
      event #31 {
        # "set bkgr-cursor back to start of the trace"
        # "get background starting from the x-position of cursor 2 until the end of trace"
        # "# of bins till end"
        # "start from this cursor\nposition"
        # "select all photons\nfrom cursor to end"
        # "add all photons"
        n203 = event-data() -> ()  [unwired: 1 in, 6 out]
        n204 = property on="MCS" class="WFGraph (strict)" props=["CrsrList", "Cursor", "Cursor Index"]() -> ("CrsrList"=w280:T15)  [unwired: 2 in, 3 out]
        n205 = property on="HH" class="Bool (strict)"() -> ("Value"=w272:bool)  [unwired: 2 in, 2 out]
        n206 = property on="auto/crossch1" class="DigNum (strict)"() -> ("Value"=w287:i32)  [unwired: 2 in, 2 out]
        n207 = case shown="False" w272 {
          tunnel: [w289 w291] -> w288
          tunnel: w287 -> [w289 w290]
          frame #0 {
          }
          frame #1 {
            n208 = Increment(x=w290) -> (x+1=w291:i32)
          }
        }
        n209 = Index Array(array=w280, index=2) -> (element=w271:T17)
        n210 = property on="binning / s" class="DigNum (strict)"() -> ("Value"=w275:dbl)  [unwired: 2 in, 2 out]
        n211 = Unbundle By Name(w271) -> ("Position.X"=w276:dbl)
        n212 = call "MCS.vi"() -> ("MCS output"=w286:T1)  [unwired: 2 in]
        n213 = Index Array(array=w286, index=w288) -> (element=w285:T18)
        n214 = Unbundle(w285) -> ("Histogram: h(x)"=w278:u32[])  [unwired: 2 out]
        n215 = Divide(x=w276, y=w275) -> (x/y=w274:dbl)
        n216 = Array Size(array=w278) -> (size(s)=w277:i32)
        n217 = Subtract(x=w277, y=w274) -> (x-y=w284:dbl)
        n218 = Array Subset(array=w278, index=w274) -> (w282:u32[])  [unwired: 1 in]
        n219 = Add Array Elements(numeric array=w282) -> (sum=w283:u32)
        n220 = Multiply(x=w284, y=w275) -> (x*y=w281:dbl)
        n221 = Divide(x=w283, y=w281) -> (x/y=w273:dbl)
        n222 = property on="B" class="DigNum (strict)"("Value"=w273) -> ()  [unwired: 2 in, 2 out]
        n223 = property on="MCS" class="WFGraph (strict)"() -> ("CrsrList"=w269:T15)  [unwired: 2 in, 2 out]
        n224 = Bundle By Name(cluster=w271, "Position.X"=0.5) -> (w268:T17)
        n225 = Replace Array Subset(array=w269, new element=w268, index=2) -> (w266:T15)
        n226 = property on="MCS" class="WFGraph (strict)"("CrsrList"=w266) -> ()  [unwired: 2 in, 2 out]
      }
      event #32 {
        n227 = event-data() -> ()  [unwired: 1 in, 5 out]
      }
      event #33 {
        n228 = event-data() -> ("NewVal"=w294:u8)  [unwired: 1 in, 4 out]
        n229 = case shown="2" w294 {
          tunnel: [u32 5 ("Numeric") u32 5 ("Numeric") u32 5 ("Numeric") u32 5 ("Numeric") u32 7 ("Numeric")] -> w293
          frame #0 {
            w295 = FALSE ("Visible")
            n230 = property on="diffusion-triplett-model" class="String"("Visible"=w295) -> ()  [unwired: 2 in, 2 out]
            n231 = property on="freeform" class="Cluster (strict)"("Visible"=w295) -> ()  [unwired: 2 in, 2 out]
            n232 = property on="Parameters 2" class="Array (strict)"("Visible"=w295) -> ()  [unwired: 2 in, 2 out]
            n233 = property on="Initial Guess Coefficient" class="Array (strict)"("Visible"=w295) -> ()  [unwired: 2 in, 2 out]
            n234 = property on="Parameters 3" class="Array (strict)"("Value"=string[] [] ("Parameters 3")) -> ()  [unwired: 2 in, 2 out]
          }
          frame #1 {
            w298 = TRUE ("Visible")
            n235 = property on="freeform" class="Cluster (strict)"("Visible"=FALSE) -> ()  [unwired: 2 in, 2 out]
            n236 = property on="Parameters 2" class="Array (strict)"("Visible"=w298) -> ()  [unwired: 2 in, 2 out]
            n237 = property on="Initial Guess Coefficient" class="Array (strict)"("Visible"=w298) -> ()  [unwired: 2 in, 2 out]
            n238 = property on="diffusion-triplett-model" class="String"("Visible"=w298) -> ()  [unwired: 2 in, 2 out]
            n239 = control-ref of="freeform"() -> (w303:refnum<vi>)
            n240 = control-ref of="Parameters 2"() -> (w301:refnum<vi>)
            n241 = control-ref of="Parameters 3"() -> (w302:refnum<vi>)
            n242 = invoke class="Clust (strict)" method="Reinit To Default"(reference=w303) -> ()  [unwired: 2 in, 3 out]
            n243 = invoke class="Arr (strict)" method="Reinit To Default"(reference=w301) -> ()  [unwired: 2 in, 3 out]
            n244 = invoke class="Arr (strict)" method="Reinit To Default"(reference=w302) -> ()  [unwired: 2 in, 3 out]
            "diffusion-triplett-model" <- "1/N*(1+(r/(1-r))*exp(-x/t1))/(1+x/t2)*(1+x/(4*t2))^(-1/2)+o"
          }
          frame #2 {
            w308 = TRUE ("Visible")
            n245 = property on="freeform" class="Cluster (strict)"("Visible"=w308) -> ()  [unwired: 2 in, 2 out]
            n246 = property on="Parameters 2" class="Array (strict)"("Visible"=w308) -> ()  [unwired: 2 in, 2 out]
            n247 = property on="Initial Guess Coefficient" class="Array (strict)"("Visible"=w308) -> ()  [unwired: 2 in, 2 out]
            n248 = Unbundle By Name("freeform") -> ("Parameters"=→"Parameters 3" →"Parameters 2":string[])
            n249 = property on="diffusion-triplett-model" class="String"("Visible"=FALSE) -> ()  [unwired: 2 in, 2 out]
          }
          frame #3 {
            w310 = FALSE ("Visible")
            n250 = property on="Parameters 3" class="Array (strict)"("Value"=string[] ["a", "b", "c"] ("Parameters 3")) -> ()  [unwired: 2 in, 2 out]
            n251 = property on="diffusion-triplett-model" class="String"("Visible"=w310) -> ()  [unwired: 2 in, 2 out]
            n252 = property on="Parameters 2" class="Array (strict)"("Visible"=w310) -> ()  [unwired: 2 in, 2 out]
            n253 = property on="Initial Guess Coefficient" class="Array (strict)"("Visible"=w310) -> ()  [unwired: 2 in, 2 out]
            n254 = property on="freeform" class="Cluster (strict)"("Visible"=w310) -> ()  [unwired: 2 in, 2 out]
          }
          frame #4 {
            w313 = FALSE ("Visible")
            n255 = property on="Fit-Type" class="Digital (strict)"("Value"=u8 0 ("Fit-Type")) -> ()  [unwired: 2 in, 2 out]
            n256 = property on="freeform" class="Cluster (strict)"("Visible"=w313) -> ()  [unwired: 2 in, 2 out]
            n257 = property on="Parameters 2" class="Array (strict)"("Visible"=w313) -> ()  [unwired: 2 in, 2 out]
            n258 = property on="Initial Guess Coefficient" class="Array (strict)"("Visible"=w313) -> ()  [unwired: 2 in, 2 out]
            n259 = property on="diffusion-triplett-model" class="String"("Visible"=w313) -> ()  [unwired: 2 in, 2 out]
            n260 = property on="Parameters 3" class="Array (strict)"("Value"=string[] [] ("Parameters 3")) -> ()  [unwired: 2 in, 2 out]
          }
        }
      }
      event #34 {
        n261 = event-data() -> ()  [unwired: 1 in, 8 out]
      }
      event #35 {
        n262 = event-data() -> ()  [unwired: 1 in, 6 out]
        n263 = property on="off times (s)" class="Array (strikt)"() -> ("Value"=w319:dbl[])  [unwired: 2 in, 2 out]
        n264 = property on="on counts" class="Array (strikt)"() -> ("Value"=w320:i32[])  [unwired: 2 in, 2 out]
        n265 = property on="intervals" class="Digital (strikt)"() -> ("Value"=w323:i32)  [unwired: 2 in, 2 out]
        n266 = call <vilib>:"Histogram.vi"("intervals"=w323, "X"=w320) -> ("X Values"=w326:dbl[], "Histogram: h(x)"=w327:i32[])  [unwired: 6 in, 2 out]
        n267 = call <vilib>:"Histogram.vi"("intervals"=w323, "X"=w319) -> ("X Values"=w324:dbl[], "Histogram: h(x)"=w325:i32[])  [unwired: 6 in, 2 out]
        n268 = Bundle("X Values"=w324, "Histogram: h(x)"=w325) -> (w321:T8)  [unwired: 1 in]
        n269 = Bundle("X Values"=w326, "Histogram: h(x)"=w327) -> (w322:T8)  [unwired: 1 in]
        n270 = property on="on count histogram" class="XYGraph (strict)"("Value"=w322) -> ()  [unwired: 2 in, 2 out]
        n271 = property on="off time histogram" class="XYGraph (strict)"("Value"=w321) -> ()  [unwired: 2 in, 2 out]
      }
      event #36 {
        n272 = event-data() -> ()  [unwired: 1 in, 6 out]
        n273 = property on="off times (s)" class="Array (strikt)"() -> ("Value"=w333:dbl[])  [unwired: 2 in, 2 out]
        n274 = property on="on counts" class="Array (strikt)"() -> ("Value"=w332:i32[])  [unwired: 2 in, 2 out]
        n275 = Bundle("Value"=w332, "Value"=w333) -> (w331:cluster{"Value":i32[], "Value":dbl[]})  [unwired: 1 in]
        n276 = stacked-sequence {
          tunnel: "Save" -> [w336 _ _]
          tunnel: w331 -> [w335 w341 w349]
          tunnel: "Open" -> [_ w342 _]
          tunnel: "Save ASCII" -> [_ _ w350]
          frame #0 {
            n277 = case shown="True" w336 {
              tunnel: w335 -> [_ w338]
              frame #0 {
              }
              frame #1 {
                n278 = call <vilib>:"Open_Create_Replace File.vi"("function (open:0)"=T9."create or replace") -> ("refnum"=w339:refnum<file>)  [unwired: 7 in, 3 out]
                n279 = Write to Binary File(file (use dialog)=w339, data=w338, 5:FALSE ("prepend array or string size? (T)")) -> ()  [unwired: 3 in, 3 out]
              }
            }
          }
          frame #1 {
            n280 = case shown="True" w342 {
              tunnel: w341 -> [_ w343]
              frame #0 {
              }
              frame #1 {
                n281 = call <vilib>:"Open_Create_Replace File.vi"("function (open:0)"=T9."open") -> ("refnum"=w346:refnum<file>)  [unwired: 7 in, 3 out]
                n282 = Read from Binary File(5:w343, 11:w346) -> (2:w348:cluster{"Value":i32[], "Value":dbl[]})  [unwired: 4 in, 3 out]
                n283 = Unbundle By Name(w348) -> ("Value"=w345:i32[], "Value"=w344:dbl[])
                n284 = property on="on counts" class="Array (strikt)"("Value"=w345) -> ()  [unwired: 2 in, 2 out]
                n285 = property on="off times (s)" class="Array (strikt)"("Value"=w344) -> ()  [unwired: 2 in, 2 out]
              }
            }
          }
          frame #2 {
            n286 = case shown="True" w350 {
              tunnel: w349 -> [_ w353]
              frame #0 {
              }
              frame #1 {
                n287 = Unbundle(w353) -> ("Value"=w352:i32[], "Value"=w351:dbl[])
                n288 = Initialize Array(0.0 ("Element")) -> (w355:dbl[][])  [unwired: 2 in]
                n289 = Insert Into Array(array=w355, new element #1=w352, new element #2=w351) -> (w354:dbl[][])  [unwired: 2 in]
                n290 = call-poly <vilib>:"Write To Spreadsheet File.vi"("2D data"=w354) -> ()  [unwired: 7 in, 1 out]
              }
            }
          }
        }
      }
      event #37 {
        n291 = event-data() -> ()  [unwired: 1 in, 6 out]
        n292 = property on="SPC Format" class="Ring (strikt)"() -> ("Value"=w358:u16)  [unwired: 2 in, 2 out]
        n293 = case shown="3" w358 {
          frame #0 {
            n294 = property on="HH" class="Boolesch (strikt)"("Value"=FALSE ("HH")) -> ()  [unwired: 2 in, 2 out]
            n295 = property on="Lifetime bins" class="Digital (strikt)"("Value"=4096 ("Lifetime bins")) -> ()  [unwired: 2 in, 2 out]
          }
          frame #1 {
          }
          frame #2 {
            n296 = property on="HH" class="Bool (strict)"("Value"=FALSE ("HH")) -> ()  [unwired: 2 in, 2 out]
            n297 = property on="Lifetime bins" class="DigNum (strict)"("Value"=4096 ("Lifetime bins")) -> ()  [unwired: 2 in, 2 out]
          }
          frame #3 {
            "HH" <- TRUE ("HH")
            "Lifetime bins" <- 32768 ("Lifetime bins")
          }
        }
      }
      event #38 {
        n298 = event-data() -> ()  [unwired: 1 in, 6 out]
        n299 = local read "areas and ratio"() -> (w372:cluster{dbl, dbl, dbl})
        n300 = local read "ratio histogram"() -> (w378:dbl[])
        n301 = Unbundle(w372) -> (w369:dbl, w365:dbl, w371:dbl)
        n302 = local read "sum high"() -> (w370:dbl)
        n303 = Insert Into Array(array=w378, new element=w371) -> (w376:dbl[])  [unwired: 1 in]
        n304 = Add(x=w369, y=w370) -> (x+y=w368:dbl)
        n305 = local write "ratio histogram"(w376) -> ()
        n306 = call <vilib>:"General Histogram.vi"("X"=w376, "max"=2.0, "min"=0.0, "# bins"=10) -> ("Histogram Graph"=→"ratio histogram":T8)  [unwired: 7 in, 4 out]
        n307 = local write "sum high"(w368) -> ()
        n308 = local read "sum low"() -> (w366:dbl)
        n309 = Add(x=w366, y=w365) -> (x+y=w367:dbl)
        n310 = local write "sum low"(w367) -> ()
      }
      event #39 {
        w382 = dbl[] [] ("X")
        n311 = event-data() -> ()  [unwired: 1 in, 6 out]
        n312 = local write "ratio histogram"(w382) -> ()
        n313 = local write "sum low"(0.0 ("sum low")) -> ()
        n314 = local write "sum high"(0.0 ("sum high")) -> ()
        n315 = call <vilib>:"General Histogram.vi"("X"=w382) -> ("Histogram Graph"=w381:T8)  [unwired: 10 in, 4 out]
        n316 = local write "ratio histogram"(w381) -> ()
      }
      event #40 {
        n317 = event-data() -> ()  [unwired: 1 in, 6 out]
        n318 = local read "ratio histogram"() -> (w390:dbl[])
        n319 = call <vilib>:"General Histogram.vi"("X"=w390, "max"=2.0, "min"=0.0, "# bins"=10) -> ("Histogram"=w389:i32[], "Axis"=w388:dbl[])  [unwired: 7 in, 3 out]
        n320 = Build Array(w388, w389) -> (w384:dbl[][])
        n321 = Transpose 2D Array(2D array=w384) -> (transposed array=w383:dbl[][])
        n322 = call-poly <vilib>:"Write To Spreadsheet File.vi"("2D data"=w383) -> ()  [unwired: 7 in, 1 out]
      }
    }
    n323 = while {
      shift-right: [w391] -> _
      shift-left: w12 -> [w395]
      shift-right: [w393] -> _
      shift-left: w10 -> [w393]
      shift-right: [w392] -> _
      shift-left: w8 -> [w392]
      stop <- w394 continue-if-true
      n324 = case shown="5" w395 {
        tunnel: [w396 w442 u32 0 ("Numeric") u32 0 ("Numeric") u32 7 ("Numeric") w716 u32 7 ("Numeric") u32 0 ("Numeric") w949 u32 7 ("Numeric") u32 7 ("Numeric")] -> w391
        tunnel: w393 -> [_ _ w498 w641 w654 _ _ _ _ _ w1013]
        tunnel: w392 -> [_ _ w497 _ w653 _ _ _ _ _ _]
        frame #0 {
          n325 = stacked-sequence {
            tunnel: [_ w405 _] -> w396
            frame #0 {
              "Busy" <- TRUE ("Busy")
            }
            frame #1 {
              n326 = call "CreateNumberedPath.vi"("File Number"="File Number", "file path"="file path") -> ("Path"=w401:path)
              n327 = case shown="3" "SPC Format" {
                tunnel: [w411 w427] -> w404
                tunnel: w401 -> [w419 w420]
                tunnel: "SPC Format" -> [_ w422]
                tunnel: [w409 w421] -> w399
                tunnel: [w407 w420] -> w398
                frame #0 {
                  n328 = call <vilib>:"Open_Create_Replace File.vi"("function (open:0)"=T9."open (read only)", "file path"=w419) -> ("file size (bytes)"=w416:i32, "new file path"=w407:path, "refnum"=w408:refnum<file>)  [unwired: 6 in, 1 out]
                  n329 = Divide(x=w416, y=u8 4) -> (x/y=w412:dbl)
                  n330 = Not Equal?(x=w407, y=path "") -> (x != y?=w413:bool)
                  n331 = Greater Than 0?(x=w412) -> (x > 0?=w414:bool)
                  n332 = Read from Binary File(5:u32 0 ("Byte-Stream-Typ"), 10:w412, 11:w408) -> (2:w410:u32[])  [unwired: 3 in, 3 out]
                  n333 = And(x=w414, y=w413) -> (x .and. y?=w411:bool)
                  n334 = call "ParseFIFO_HH.vi"("RawData"=w410) -> ("RawData Out"=w409:T19)  [unwired: 1 in]
                }
                frame #1 {
                  n335 = call "Read From I16 File.vi"("file path (dialog if empty)"=w420) -> ("mark after read (bytes)"=w428:i32, "1D array"=w423:i16[], "new file path (Not A Path if cancelled)"=w429:path)  [unwired: 6 in, 2 out]
                  n336 = Not Equal?(x=w429, y=path "") -> (x != y?=w425:bool)
                  n337 = Greater Than 0?(x=w428) -> (x > 0?=w426:bool)
                  n338 = And(x=w426, y=w425) -> (x .and. y?=w427:bool)
                  n339 = To Unsigned Word Integer(number=w423) -> (unsigned 16bit integer=w424:u16[])
                  n340 = call "ParseFIFO.vi"("SPC Format"=w422, "FIFO rawdata"=w424) -> ("rawdata"=w421:T20)
                }
              }
              n341 = case shown="True" w404 {
                tunnel: [0 1] -> w405
                tunnel: w399 -> [_ w433]
                frame #0 {
                }
                frame #1 {
                  n342 = Unbundle By Name(w433) -> ("router channels"=w432:u8[], "invalid times"=w436:u32[], "gap times"=w435:u32[])
                  n343 = Array Size(array=w432) -> (size(s)=→"all photons":i32)
                  n344 = Array Size(array=w436) -> (size(s)=→"invalid":i32)
                  n345 = Array Size(array=w435) -> (size(s)=→"gaps":i32)
                  n346 = call "Rawdata.vi"("input rawdata"=w433, "set"=TRUE) -> ()  [unwired: 1 out]
                }
              }
              n347 = property on="file path" class="Path"("Value"=w398) -> ()  [unwired: 2 in, 2 out]
            }
            frame #2 {
              n348 = local write "Busy"(FALSE ("Busy")) -> ()
            }
          }
        }
        frame #1 {
          n349 = stacked-sequence {
            tunnel: [_ w445 _] -> w442
            frame #0 {
              n350 = local write "Busy"(TRUE ("Busy")) -> ()
            }
            frame #1 {
              n351 = call "Rawdata.vi"() -> ("output rawdata"=w444:T16)  [unwired: 2 in]
              n352 = stacked-sequence {
                seq-local: [w447 _] -> [_ w477]
                seq-local: [w448 _] -> [_ w478]
                seq-local: [w446 _] -> [_ w475]
                tunnel: [_ u32 8 ("Numeric")] -> w445
                tunnel: w444 -> [w464 _]
                frame #0 {
                  n353 = property on="HH" class="Boolesch (strikt)"() -> ("Value"=w446:bool)  [unwired: 2 in, 2 out]
                  n354 = case shown="False" w446 {
                    tunnel: "binning / s" -> [w473 _]
                    tunnel: w464 -> [w471 _]
                    tunnel: [w470 _] -> w448
                    tunnel: [w469 _] -> w447
                    frame #0 {
                      n355 = Unbundle By Name(w471) -> ("invalid times"=w472:u32[], "gap times"=w474:u32[])
                      n356 = call "SummarizeFIFOTimes.vi"("binning (s)"=w473, "macro times (s)"=w472) -> ("MCS"=w470:T21)
                      n357 = call "SummarizeFIFOTimes.vi"("binning (s)"=w473, "macro times (s)"=w474) -> ("MCS"=w469:T21)
                    }
                    frame #1 {
                    }
                  }
                  n358 = Build Array("Donor", "Transmitter 1", "Transmitter 2", "Acceptor") -> (→"channels":u8[])
                  n359 = call "BinFIFO.vi"("HydraHarp"=w446, "binning (s)"="binning / s", "rawdata"=w464) -> ("Counts"=w468:u32[], "MCS"=w462:u32[][])
                  n360 = Index Array(array=w468, index #1="Donor", index #2="Transmitter 1", index #3="Transmitter 2", index #4="Acceptor") -> (element #1=→"donor":u32, element #2=→"T1":u32, element #3=→"T 2":u32, element #4=→"element":u32)
                  n361 = call "ClusterFourChannels.vi"("Trace3"="Acceptor", "binning (s)"="binning / s", "Trace 2"="Transmitter 2", "Trace 1"="Transmitter 1", "Trace 0"="Donor", "MCS"=w462) -> ("channel 3"=w450:cluster{i32, "binning (s)":dbl, "MCS":u32[]}, "channel 2"=w459:T22, "channel 1"=w458:T22, "channel 0"=w457:T22, "sum"=w456:T22)
                  n362 = Build Array(w456, w457, w458, w459, w450, w448, w447) -> (w449:T23)
                  "MCS" <- w449
                  n363 = call "MCS.vi"("MCS input"=w449, "set"=TRUE) -> ()  [unwired: 1 out]
                }
                frame #1 {
                  n364 = case shown="False" w475 {
                    tunnel: w478 -> [w483 _]
                    tunnel: w477 -> [w480 _]
                    frame #0 {
                      n365 = Unbundle By Name(w483) -> ("Histogram: h(x)"=w481:i32[])
                      n366 = Unbundle By Name(w480) -> ("Histogram: h(x)"=w482:i32[])
                      n367 = Array Max & Min(array=w481) -> (max value=w485:i32)  [unwired: 3 out]
                      n368 = Array Max & Min(array=w482) -> (max value=w484:i32)  [unwired: 3 out]
                      n369 = Max & Min(x=w485, y=w484) -> (max(x,y)=w486:i32)  [unwired: 1 out]
                      n370 = case shown="True" "Case Constant\n(See Context Help)" {
                        tunnel: w486 -> [_ w491]
                        frame #0 {
                        }
                        frame #1 {
                          n371 = Multiply(x=w491, y=5) -> (x*y=w488:i32)
                          n372 = control-ref of="MCS"() -> (w487:refnum<vi>)
                          n373 = call "SetScale.vi"("max"=w488, "min"=u32 0 ("Y Scale.Range:Minimum"), "Active Y Scale"=1, "reference"=w487) -> ()
                        }
                      }
                    }
                    frame #1 {
                    }
                  }
                }
              }
            }
            frame #2 {
              n374 = local write "Busy"(FALSE ("Busy")) -> ()
            }
          }
        }
        frame #2 {
          n375 = local read "HH Binning / TAC Gain"() -> (w503:u16)
          n376 = local read "histogram lenght (µs)"() -> (w502:dbl)
          n377 = local read "delay channel 1"() -> (w501:bool)
          n378 = local read "center peak (µs)"() -> (w500:dbl)
          n379 = local read "lateral peaks"() -> (w499:u32)
          n380 = local read "TAC range (ns)"() -> (w495:dbl)
          n381 = local read "rebinning"() -> (w504:u16)
          n382 = local read "Lifetime bins"() -> (w496:i32)
          n383 = local read "HH"() -> (w494:bool)
          n384 = call "Rawdata.vi"() -> ("output rawdata"=w505:T16)  [unwired: 2 in]
          n385 = case shown="1" "binning type" {
            tunnel: "binning" -> [w526 w591]
            tunnel: w505 -> [w527 w592]
            tunnel: w504 -> [w525 w588]
            tunnel: w503 -> [w524 w589]
            tunnel: w502 -> [w523 w583]
            tunnel: w501 -> [w522 w587]
            tunnel: w500 -> [w521 w582]
            tunnel: w499 -> [w520 w584]
            tunnel: w498 -> [_ _]
            tunnel: w497 -> [w511 w577]
            tunnel: w496 -> [_ w576]
            tunnel: w495 -> [w509 w575]
            tunnel: w494 -> [w510 w574]
            frame #0 {
              n386 = stacked-sequence {
                tunnel: w527 -> [w537 w548 w571]
                tunnel: w526 -> [w536 w545 w562]
                tunnel: [w535 _ _] -> w519
                tunnel: w525 -> [_ w547 _]
                tunnel: w524 -> [_ w546 _]
                tunnel: [_ w544 _] -> w518
                tunnel: w523 -> [_ _ w570]
                tunnel: w522 -> [_ _ w569]
                tunnel: w521 -> [_ _ w567]
                tunnel: w520 -> [_ _ w566]
                tunnel: [_ _ w565] -> w517
                tunnel: [_ _ w561] -> w514
                tunnel: w511 -> [_ w543 _]
                tunnel: w510 -> [_ w542 _]
                tunnel: w509 -> [_ w541 _]
                frame #0 {
                  n387 = property on="Acceptor" class="DigNum (strict)"() -> ("Value"=w529:u8)  [unwired: 2 in, 2 out]
                  n388 = property on="HH" class="Boolesch (strikt)"() -> ("Value"=w528:bool)  [unwired: 2 in, 2 out]
                  n389 = call "BinFIFO.vi"("HydraHarp"=w528, "binning (s)"=w536, "rawdata"=w537) -> ("MCS"=w534:u32[][])  [unwired: 1 out]
                  n390 = property on="Donor" class="Digital (strict)"() -> ("Value"=w530:u8)  [unwired: 2 in, 2 out]
                  n391 = Index Array(array=w534, index (row) #1=w529, index (row) #2=w530) -> (element #1=w531:u32[], element #2=w533:u32[])  [unwired: 2 in]
                  n392 = Add(x=w531, y=w533) -> (x+y=w532:u32[])
                  n393 = Divide(x=w531, y=w532) -> (x/y=w538:dbl[])
                  n394 = Bundle(0.0, "binning"=w536, w538) -> (w535:cluster{dbl, "binning":dbl, dbl[]})  [unwired: 1 in]
                }
                frame #1 {
                  n395 = local read "Lifetime bins"() -> (w540:i32)
                  n396 = Divide(x=w540, y=w547) -> (x/y=w551:dbl)
                  n397 = Round Toward +Infinity(x=w551) -> (ceil(x): smallest int >= x=w553:dbl)
                  n398 = case shown="True" w542 {
                    tunnel: w553 -> [w556 w560]
                    tunnel: [w554 w559] -> w552
                    tunnel: w546 -> [w557 w558]
                    tunnel: w541 -> [w555 _]
                    frame #0 {
                      n399 = call "CalcChannelWidth.vi"("TAC gain"=w557, "channel count"=w556, "TAC window (ns)"=w555) -> ("channel width (ns)"=w554:dbl)
                    }
                    frame #1 {
                      n400 = call "CalcChannelWidth_HH.vi"("HH binning"=w558, "channel count"=w560) -> ("channel width (ns)"=w559:dbl)  [unwired: 1 in]
                    }
                  }
                  n401 = call "BinMLE.vi"("channel width (ns)"=w552, "channel count"=w540, "rebinning"=w547, "binning"=w545, "input range"=w543, "rawdata"=w548) -> ("MLE trace"=w550:dbl[])
                  n402 = Bundle(0.0, "binning"=w545, "MLE trace"=w550) -> (w544:cluster{dbl, "binning":dbl, "MLE trace":dbl[]})  [unwired: 1 in]
                }
                frame #2 {
                  n403 = Boolean To (0,1)(Boolean=w569) -> (0, 1=w568:i16)
                  n404 = call "BinCoincidence.vi"("lateral peaks"=w566, "rawdata"=w571, "center peak (µs)"=w567, "delay channel"=w568, "histogram lenght (µs)"=w570, "binning"=w562) -> ("center peak trace"=w563:u32[], "coincidence trace"=w573:dbl[])
                  n405 = Bundle(0.0, "binning"=w562, "coincidence trace"=w573) -> (w565:T24)  [unwired: 1 in]
                  n406 = Bundle(0.0, "binning"=w562, "center peak trace"=w563) -> (w561:T25)  [unwired: 1 in]
                }
              }
              n407 = property on="traces" class="XYGraph (strict)"("Visible"=FALSE) -> ()  [unwired: 2 in, 2 out]
              n408 = property on="traces" class="WaveformGraph (strict)"("Visible"=TRUE) -> ()  [unwired: 2 in, 2 out]
              n409 = Build Array(w519, w518, w517, w514) -> (w512:T26)
              "traces" <- w512
              n410 = call "BinningTraces.vi"("binned traces in"=w512, "set"=TRUE) -> ()  [unwired: 1 out]
            }
            frame #1 {
              n411 = stacked-sequence {
                tunnel: w592 -> [w603 w613 w636]
                tunnel: w591 -> [w601 w615 w633]
                tunnel: "shift (photons)" -> [w602 w614 w634]
                tunnel: w589 -> [_ w616 _]
                tunnel: w588 -> [_ w611 _]
                tunnel: w587 -> [_ _ w638]
                tunnel: [_ w608 _] -> w585
                tunnel: [w595 _ _] -> w586
                tunnel: w584 -> [_ _ w635]
                tunnel: w583 -> [_ _ w632]
                tunnel: w582 -> [_ _ w631]
                tunnel: [_ _ w628] -> w581
                tunnel: [_ _ w626] -> w580
                tunnel: w577 -> [_ w607 _]
                tunnel: w576 -> [_ w606 _]
                tunnel: w575 -> [_ w605 _]
                tunnel: w574 -> [_ w604 _]
                frame #0 {
                  n412 = call "SlideFIFO.vi"("shift (photons)"=w602, "window (photons)"=w601, "rawdata"=w603) -> ("SlideTime"=w597:dbl[], "SlideMCS"=w599:u32[][])
                  n413 = Index Array(array=w599, index (row)=1) -> (element=w598:u32[])  [unwired: 1 in]
                  n414 = Divide(x=w598, y=w601) -> (x/y=w596:dbl[])
                  n415 = Bundle("SlideTime"=w597, w596) -> (w595:cluster{"SlideTime":dbl[], dbl[]})  [unwired: 1 in]
                }
                frame #1 {
                  n416 = Divide(x=w606, y=w611) -> (x/y=w617:dbl)
                  n417 = Round Toward +Infinity(x=w617) -> (ceil(x): smallest int >= x=w618:dbl)
                  n418 = case shown="False" w604 {
                    tunnel: w618 -> [w621 w625]
                    tunnel: w616 -> [w622 w624]
                    tunnel: [w619 w623] -> w612
                    tunnel: w605 -> [w620 _]
                    frame #0 {
                      n419 = call "CalcChannelWidth.vi"("TAC gain"=w622, "channel count"=w621, "TAC window (ns)"=w620) -> ("channel width (ns)"=w619:dbl)
                    }
                    frame #1 {
                      n420 = call "CalcChannelWidth_HH.vi"("HH binning"=w624, "channel count"=w625) -> ("channel width (ns)"=w623:dbl)  [unwired: 1 in]
                    }
                  }
                  n421 = call "SlideLifetime.vi"("rawdata"=w613, "window (photons)"=w615, "input range"=w607, "channel count"=w606, "rebinning"=w611, "channel width (ns)"=w612, "shift (photons)"=w614) -> ("SlideLifetime"=w609:dbl[], "SlideTime"=w610:dbl[])
                  n422 = Bundle("SlideTime"=w610, "SlideLifetime"=w609) -> (w608:T27)  [unwired: 1 in]
                }
                frame #2 {
                  n423 = Boolean To (0,1)(Boolean=w638) -> (0, 1=w637:i16)
                  n424 = call "SlideCoincidence.vi"("shift (photons)"=w634, "lateral peaks"=w635, "window (photons)"=w633, "center peak (µs)"=w631, "delay channel"=w637, "histogram lenght (µs)"=w632, "rawdata"=w636) -> ("SlideTime"=w629:dbl[], "SlideCoincidence"=w630:dbl[], "SlideCenterPeak"=w627:u32[])
                  n425 = Bundle("SlideTime"=w629, "SlideCoincidence"=w630) -> (w628:T28)  [unwired: 1 in]
                  n426 = Bundle("SlideTime"=w629, "SlideCenterPeak"=w627) -> (w626:T29)  [unwired: 1 in]
                }
              }
              n427 = property on="traces" class="WaveformGraph (strict)"("Visible"=TRUE) -> ()  [unwired: 2 in, 2 out]
              n428 = property on="traces" class="XYGraph (strict)"("Visible"=TRUE) -> ()  [unwired: 2 in, 2 out]
              n429 = Build Array(w586, w585, w581, w580) -> (w578:T30)
              "traces" <- w578
              n430 = call "SlidingTraces.vi"("sliding traces in"=w578, "set"=TRUE) -> ()  [unwired: 1 out]
            }
          }
        }
        frame #3 {
          n431 = Boolean To (0,1)(Boolean="delay channel 1") -> (0, 1=w649:i16)
          n432 = call "Rawdata.vi"() -> ("output rawdata"=w644:T16)  [unwired: 2 in]
          n433 = call "CoincidenceHist.vi"("delayed channel"=w649, "length (µs)"="histogram lenght (µs)", "range"=w641, "input rawdata"=w644) -> ("coincidence histogram"=w642:T12)
          "coincidence histogram" <- w642
          n434 = Unbundle By Name(w642) -> ("histogram"=w640:u32[])
          n435 = call "CoincidenceHistogram.vi"("coincidence histogram in"=w642, "set"=TRUE) -> ()  [unwired: 1 out]
          n436 = Add Array Elements(numeric array=w640) -> (sum=→"sum":u32)
          n437 = call "GetCoincidenceRatio.vi"("lateral peaks"="lateral peaks", "center peak (µs)"="center peak (µs)", "histogram"=w640) -> ("coincidence ratio"=→"coincidence ratio":dbl)
        }
        frame #4 {
          n438 = stacked-sequence {
            tunnel: w654 -> [w676 _]
            tunnel: w653 -> [_ w704]
            frame #0 {
              w685 = 0.0
              n439 = property on="Lifetime bins" class="Digital (strikt)"() -> ("Value"=w674:i32)  [unwired: 2 in, 2 out]
              n440 = property on="HH" class="Boolesch (strikt)"() -> ("Value"=w661:bool)  [unwired: 2 in, 2 out]
              n441 = call "Rawdata.vi"() -> ("output rawdata"=w669:T16)  [unwired: 2 in]
              n442 = Divide(x=w674, y="rebinning") -> (x/y=w678:dbl)
              n443 = Round Toward +Infinity(x=w678) -> (ceil(x): smallest int >= x=w677:dbl)
              n444 = case shown="False" w661 {
                tunnel: "HH Binning / TAC Gain" -> [w698 w702]
                tunnel: w677 -> [w697 w701]
                tunnel: [w695 w700] -> w665
                tunnel: "TAC range (ns)" -> [w696 _]
                tunnel: "rebinning" -> [_ w699]
                frame #0 {
                  n445 = call "CalcChannelWidth.vi"("TAC gain"=w698, "channel count"=w697, "TAC window (ns)"=w696) -> ("channel width (ns)"=w695:dbl)
                }
                frame #1 {
                  n446 = call "CalcChannelWidth_HH.vi"("HH binning"=w702, "channel count"=w701, "rebinning"=w699) -> ("channel width (ns)"=w700:dbl)
                }
              }
              n447 = call "FIFOLifetime_HH.vi"("input rawdata"=w669, "range"=w676, "rebinning"="rebinning", "channel count"=w674) -> ("lifetime histograms"=w680:u32[][])  [unwired: 1 in]
              n448 = call "DecayCluster2.vi"("lifetime histograms"=w680, "ch1 (0=sum)"="ch1 (0=sum)", "channel width (ns)"=w665, "ch2"="ch2", "ch3"="ch3") -> ("lifetime histograms"=w659:T14)
              n449 = Unbundle By Name(w659) -> ("sum"=w664:u32[], "channel 0"=w663:u32[], "channel 1"=w662:u32[])
              n450 = Unbundle(w669) -> ("macro times"=w668:dbl[])  [unwired: 4 out]
              n451 = case shown="False" w661 {
                tunnel: [w690 w694] -> w658
                tunnel: w664 -> [w691 w694]
                tunnel: w663 -> [w686 w693]
                tunnel: [w687 w693] -> w657
                tunnel: w662 -> [w689 w692]
                tunnel: [w688 w692] -> w656
                frame #0 {
                  n452 = Reverse 1D Array(array=w686) -> (reversed array=w687:u32[])
                  n453 = Reverse 1D Array(array=w689) -> (reversed array=w688:u32[])
                  n454 = Reverse 1D Array(array=w691) -> (reversed array=w690:u32[])
                }
                frame #1 {
                }
              }
              n455 = Array Max & Min(array=w668) -> (max value=→"max value":dbl)  [unwired: 3 out]
              n456 = Bundle By Name(cluster=w659, "sum"=w658, "channel 0"=w657, "channel 1"=w656) -> (w655:T14)
              n457 = Add Array Elements(numeric array=w656) -> (sum=→"selected photons ch3":u32)
              n458 = Bundle(w685, "channel width (ns)"=w665, "sum"=w658) -> (w683:T31)  [unwired: 1 in]
              n459 = Bundle(w685, "channel width (ns)"=w665, "channel 0"=w657) -> (w682:T32)  [unwired: 1 in]
              n460 = Bundle(w685, "channel width (ns)"=w665, "channel 1"=w656) -> (w681:T33)  [unwired: 1 in]
              n461 = call "LifetimeHistograms.vi"("input lifetime histograms"=w655, "set"=TRUE) -> ()  [unwired: 1 out]
              n462 = Build Array(w683, w682, w681) -> (→"lifetime histogram":T4)
            }
            frame #1 {
              n463 = case shown="True" "Case Constant\n(See Context Help) 2" {
                tunnel: w704 -> [_ w705]
                frame #0 {
                }
                frame #1 {
                  n464 = call "LifetimeHistograms.vi"() -> ("output lifetime histograms"=w710:T14)  [unwired: 2 in]
                  n465 = Unbundle By Name(w710) -> ("sum"=w708:u32[], "channel 0"=w707:u32[], "channel 1"=w706:u32[], "channel width (ns)"=w709:dbl)
                  n466 = call "MLE.vi"("input range"=w705, "channel width (ns)"=w709, "lifetime histograms"=w708) -> ("lifetime (ns)"=w715:dbl[])
                  n467 = call "MLE.vi"("input range"=w705, "channel width (ns)"=w709, "lifetime histograms"=w707) -> ("lifetime (ns)"=w714:dbl[])
                  n468 = call "MLE.vi"("input range"=w705, "channel width (ns)"=w709, "lifetime histograms"=w706) -> ("lifetime (ns)"=w713:dbl[])
                  n469 = Build Array(w715, w714, w713) -> (w712:dbl[][])
                  n470 = Transpose 2D Array(2D array=w712) -> (transposed array=→"lifetime (ns)":dbl[][])
                }
              }
            }
          }
        }
        frame #5 {
          n471 = stacked-sequence {
            tunnel: [_ _ u32 7 ("Numeric") _] -> w716
            frame #0 {
              n472 = local write "Busy"(TRUE ("Busy")) -> ()
            }
            frame #1 {
              w754 = u32 2 ("Cursor.Cursor Locked")
              w749 = TRUE ("Cursor.Allow Drag")
              n473 = property on="MCS" class="WaveformGraph (strict)"("Active Cursor"=u32 0, "Cursor.Cursor Lock Style"=w754, "Cursor.Allow Drag"=w749, "Active Cursor"=u32 1, "Cursor.Cursor Lock Style"=w754, "Cursor.Allow Drag"=w749) -> ("Cursor.Cursor Index"=w753:i32, "Cursor.Cursor Index"=w750:i32)  [unwired: 2 in, 2 out]
              n474 = call "MCS.vi"() -> ("MCS output"=w726:T1)  [unwired: 2 in]
              n475 = Max & Min(x=w753, y=w750) -> (max(x,y)=w724:i32, min(x,y)=w744:i32)
              n476 = Index Array(array=w726, index=0) -> (element=w725:T18)
              n477 = Subtract(x=w724, y=w744) -> (x-y=w720:i32)
              n478 = Unbundle(w725) -> ("Histogram: h(x)"=w728:u32[])  [unwired: 2 out]
              n479 = To Unsigned Long Integer(number=w728) -> (unsigned 32bit integer=w729:u32[])
              n480 = Array Subset(array=w729, index=w744, length=w720) -> (w723:u32[])
              n481 = Add Array Elements(numeric array=w723) -> (sum=w722:u32)
              n482 = Array Max & Min(array=w723) -> (max value=w733:u32, min value=w730:u32)  [unwired: 2 out]
              n483 = property on="binning / s" class="Digital (strict)"() -> ("Value"=w719:dbl)  [unwired: 2 in, 2 out]
              n484 = Multiply(x=w719, y=w720) -> (x*y=w721:dbl)
              n485 = Divide(x=w722, y=w721) -> (x/y=→"Mean Intensity/\nbackground":dbl)
              n486 = Subtract(x=w733, y=w730) -> (x-y=w731:u32)
              n487 = Increment(x=w731) -> (x+1=w732:u32)
              n488 = property on="Int Histogram" class="XYGraph (strict)"("Active Cursor"=u32 0, "Cursor.Cursor Lock Style"=u32 0 ("Cursor.Cursor Locked"), "Cursor.Cursor Position:Cursor X"="Int-Threshold") -> ()  [unwired: 2 in, 2 out]
              n489 = call "on-off-hist.vi"("Array"=w723, "Data bin time"=w719, "Threshold"="Int-Threshold", "Threshold 2"="Int-Threshold 2") -> ("0n 2"=→"on2":cluster{"Axis":dbl[], "Histogram":i32[]}, "Avg off"=→"Avg off":dbl, "Avg On"=→"Avg On":dbl, "On plot 1"=→"On plot1":cluster{"Axis":dbl[], "Histogram":i32[]}, "Offs 0"=→"Offs 0":cluster{"Axis":dbl[], "Histogram":i32[]})  [unwired: 2 out]
              n490 = Divide(x=w732, y=2.0) -> (x/y=w748:dbl)
              n491 = call <vilib>:"General Histogram.vi"("X"=w723, "max"=w733, "min"=w730, "# bins"=w748) -> ("Histogram"=w734:i32[], "Axis"=w735:dbl[])  [unwired: 7 in, 3 out]
              n492 = Bundle("Axis"=w735, "Histogram"=w734) -> (→"Int Histogram":cluster{"Axis":dbl[], "Histogram":i32[]})  [unwired: 1 in]
            }
            frame #2 {
              n493 = property on="none/auto/cross" class="Digital (strict)"() -> ("Value"=w755:u8)  [unwired: 2 in, 2 out]
              n494 = case shown="1" w755 {
                frame #0 {
                }
                frame #1 {
                  w761 = cluster{dbl[], "Best Fit":dbl[]}[] [] ("Autocorr 2")
                  n495 = for {
                    N: 1 -> [_]
                    shift-right: [w798] -> w758
                    shift-left: w761 -> [w795]
                    tunnel: [w797] -> w764 mode=indexing
                    tunnel: [w796] -> w763 mode=indexing
                    shift-right: [w793] -> w759
                    shift-left: dbl[][] [] -> [w792]
                    shift-right: [w788] -> w757
                    shift-left: w761 -> [w786]
                    w816 = u32 2 ("Write Attribute")
                    w828 = TRUE ("Write Attribute")
                    n496 = property on="auto/crossch1" class="Digital (strict)"() -> ("Value"=w780:i32)  [unwired: 2 in, 2 out]
                    n497 = call "Rawdata.vi"() -> ("output rawdata"=w803:T16)  [unwired: 2 in]
                    n498 = property on="channels" class="Array (strict)"() -> ("Value"=w800:u8[])  [unwired: 2 in, 2 out]
                    n499 = Unbundle By Name(w803) -> ("router channels"=w804:u8[], "macro times"=w805:dbl[])
                    n500 = Increment(x=w780) -> (x+1=w779:i32)
                    n501 = property on="MCS" class="WFGraph (strict)"("Active Cursor"=u32 0, "Cursor.Cursor Lock Style"=w816, "Cursor.Allow Drag"=w828, "Active Cursor"=u32 1, "Cursor.Cursor Lock Style"=w816, "Cursor.Allow Drag"=w828) -> ("Cursor.Cursor Index"=w827:i32, "Cursor.Cursor Index"=w826:i32)  [unwired: 2 in, 2 out]
                    n502 = Index Array(array=w800, index=w780) -> (element=w778:u8)
                    n503 = property on="HH" class="Boolesch (strikt)"() -> ("Value"=w781:bool)  [unwired: 2 in, 2 out]
                    n504 = call "MCS.vi"() -> ("MCS output"=w813:T1)  [unwired: 2 in]
                    n505 = Decrement(x=w778) -> (x-1=w783:u8)
                    n506 = Index Array(array=w813, index=w779) -> (element=w831:T18)
                    n507 = Select(t=w778, s=w781, f=w783) -> (s? t:f=w782:u8)
                    n508 = call <vilib>:"General Histogram.vi"("X"=w804, "max"=10.5, "min"=-0.5, "# bins"=11) -> ("Histogram"=w808:i32[], "Axis"=w810:dbl[])  [unwired: 7 in, 3 out]
                    n509 = Max & Min(x=w827, y=w826) -> (max(x,y)=w825:i32, min(x,y)=w822:i32)
                    n510 = property on="binning / s" class="DigNum (strict)"() -> ("Value"=w771:dbl)  [unwired: 2 in, 2 out]
                    n511 = Unbundle(w831) -> ("Histogram: h(x)"=w784:u32[])  [unwired: 2 out]
                    n512 = Subtract(x=w825, y=w822) -> (x-y=w772:i32)
                    n513 = Index Array(array=w808, index=w782) -> (element=w807:i32)
                    n514 = Bundle("Axis"=w810, "Histogram"=w808) -> (→"ChannelsHist":cluster{"Axis":dbl[], "Histogram":i32[]})  [unwired: 1 in]
                    n515 = Array Subset(array=w784, index=0, length=w822) -> (w824:u32[])
                    n516 = Array Subset(array=w784, index=w822, length=w772) -> (w829:u32[])
                    n517 = Equal To 0?(x=w778) -> (x = 0?=w799:bool)
                    n518 = property on="B" class="DigNum (strict)"() -> ("Value"=w773:dbl)  [unwired: 2 in, 2 out]
                    n519 = Add Array Elements(numeric array=w824) -> (sum=w818:u32)
                    n520 = Add Array Elements(numeric array=w829) -> (sum=w769:u32)
                    n521 = property on="freeform" class="Cluster (strict)"() -> ("Value"=w790:T5)  [unwired: 2 in, 2 out]
                    n522 = Multiply(x=w772, y=w771) -> (x*y=w770:dbl)
                    n523 = Initialize Array(0 ("element"), w807) -> (w801:i32[])
                    n524 = local read "skip"() -> (w765:i32)
                    n525 = Divide(x=w769, y=w770) -> (x/y=w768:dbl)
                    n526 = case shown="False" w799 {
                      tunnel: w805 -> [w838 w855]
                      tunnel: w801 -> [w837 _]
                      tunnel: w782 -> [w833 _]
                      tunnel: w804 -> [w836 _]
                      tunnel: [w834 w854] -> w785
                      frame #0 {
                        n527 = for {
                          tunnel: w838 -> [w841] mode=indexing
                          shift-right: [w842] -> w835
                          shift-left: w837 -> [w843]
                          tunnel: w833 -> [w845]
                          tunnel: w836 -> [w844] mode=indexing
                          shift-right: [w839] -> _
                          shift-left: u32 0 ("element") -> [w840]
                          n528 = Equal?(x=w844, y=w845) -> (x = y?=w846:bool)
                          n529 = case shown="True" w846 {
                            tunnel: w843 -> [w848 w853]
                            tunnel: [w848 w852] -> w842
                            tunnel: w841 -> [_ w851]
                            tunnel: w840 -> [w847 w849]
                            tunnel: [w847 w850] -> w839
                            frame #0 {
                            }
                            frame #1 {
                              n530 = Replace Array Subset(array=w853, new element=w851, index=w849) -> (w852:i32[])
                              n531 = Increment(x=w849) -> (x+1=w850:u32)
                            }
                          }
                        }
                        n532 = To Long Integer(number=w835) -> (32bit integer=w834:i32[])
                      }
                      frame #1 {
                        n533 = To Long Integer(number=w855) -> (32bit integer=w854:i32[])
                      }
                    }
                    n534 = Array Subset(array=w785, index=w818, length=w769) -> (w820:i32[])
                    n535 = Index Array(array=w820, index=0 ("Index")) -> (element=w819:i32)
                    n536 = property on="biExp fit" class="Bool (strict)"() -> ("Value"=w767:bool)  [unwired: 2 in, 2 out]
                    n537 = Subtract(x=w820, y=w819) -> (x-y=w817:i32[])
                    n538 = property on="S+B (Hz)" class="DigNum (strict)"("Value"=w768) -> ()  [unwired: 2 in, 2 out]
                    n539 = call "Autocorr_sub.vi"("Freeform"=w790, "skip"=w765, "min bin time (ns)"="min bin time (ns)", "MacroTimes"=w817, "Initial Guess Coefficient"="Initial Guess Coefficient", "Fit-Type"="Fit-Type") -> ("off"=w796:dbl, "on"=w797:dbl, "Autocorr 2"=w777:cluster{dbl[], "Best Fit":dbl[]}[], "Deviation"=w787:cluster{dbl[], dbl[]}, "Best Fit Coefficients"=w791:dbl[])  [unwired: 1 in]
                    n540 = Build Array (concatenate)(w792, w791) -> (w793:dbl[][])
                    n541 = call "2exp fit cs.vi"("S+B"=w768, "biExp fit"=w767, "B"=w773, "Autocorr data"=w777) -> ("best fit"=w775:dbl[], "results"=w766:cluster{dbl, dbl, dbl, dbl, dbl, dbl}, "x-values"=w776:dbl[])  [unwired: 2 in]
                    n542 = Bundle("x-values"=w776, "best fit"=w775) -> (w774:cluster{"x-values":dbl[], "best fit":dbl[]})  [unwired: 1 in]
                    n543 = property on="results" class="Clust (strict)"("Value"=w766) -> ()  [unwired: 2 in, 2 out]
                    n544 = Build Array (concatenate)(w795, w777, w774) -> (w798:cluster{"x-values":dbl[], "best fit":dbl[]}[])
                    n545 = Build Array (concatenate)(w787, w786) -> (w788:cluster{dbl[], "Best Fit":dbl[]}[])
                  }
                  "on" <- w764
                  "off" <- w763
                  "Best Fit Coefficient" <- w759
                  "Autocorrelation" <- w758
                  "Deviation" <- w757
                }
                frame #2 {
                  n546 = call "Rawdata.vi"() -> ("output rawdata"=w893:T16)  [unwired: 2 in]
                  n547 = property on="auto/crossch1" class="Digital (strict)"() -> ("Value"=w884:i32)  [unwired: 2 in, 2 out]
                  n548 = property on="hardware channels" class="Array (strict)"() -> ("Value"=w865:u8[])  [unwired: 2 in, 2 out]
                  n549 = Unbundle By Name(w893) -> ("router channels"=w876:u8[], "macro times"=w868:dbl[])
                  n550 = To Double Precision Float(number=w865) -> (double precision float=w864:dbl[])
                  n551 = property on="HH" class="Boolesch (strikt)"() -> ("Value"=w878:bool)  [unwired: 2 in, 2 out]
                  n552 = Index Array(array=w864, index #1=w884, index #2="cross ch2") -> (element #1=w867:dbl, element #2=w866:dbl)
                  n553 = Decrement(x=w876) -> (x-1=w877:u8[])
                  n554 = Decrement(x=w867) -> (x-1=w858:dbl)
                  n555 = Decrement(x=w866) -> (x-1=w857:dbl)
                  n556 = Select(t=w877, s=w878, f=w876) -> (s? t:f=w875:u8[])
                  n557 = call <vilib>:"General Histogram.vi"("X"=w875, "max"=10.5, "min"=-0.5, "# bins"=11) -> ("Histogram"=w861:i32[], "Axis"=w862:dbl[])  [unwired: 7 in, 3 out]
                  n558 = Less Than 0?(x=w857) -> (x < 0?=w856:bool)
                  n559 = Less Than 0?(x=w858) -> (x < 0?=w859:bool)
                  n560 = case shown="False" w859 {
                    tunnel: [w903 w904] -> w890
                    tunnel: w861 -> [w902 w905]
                    tunnel: w858 -> [w901 _]
                    frame #0 {
                      n561 = Index Array(array=w902, index=w901) -> (element=w903:i32)
                    }
                    frame #1 {
                      n562 = Add Array Elements(numeric array=w905) -> (sum=w904:i32)
                    }
                  }
                  n563 = case shown="False" w856 {
                    tunnel: [w898 w899] -> w889
                    tunnel: w857 -> [w897 _]
                    tunnel: w861 -> [w896 w900]
                    frame #0 {
                      n564 = Index Array(array=w896, index=w897) -> (element=w898:i32)
                    }
                    frame #1 {
                      n565 = Add Array Elements(numeric array=w900) -> (sum=w899:i32)
                    }
                  }
                  n566 = Initialize Array(0 ("element"), w889) -> (w888:i32[])
                  n567 = Initialize Array(0 ("element"), w890) -> (w892:i32[])
                  n568 = control-ref of="binning / s"() -> (w871:refnum<vi>)
                  n569 = To Long Integer(number=w868) -> (32bit integer=w874:i32[])
                  n570 = control-ref of="MCS"() -> (w872:refnum<vi>)
                  n571 = call "selectByTime.vi"("0-array (ch1 length)"=w892, "router channels"=w875, "macro times"=w874, "0-array (ch2 length)"=w888, "Cross Ch2 (hardware)"=w857, "Cross Ch1 (hardware)"=w858) -> ("macro times ch2"=w886:i32[], "macro times ch1"=w891:i32[])  [unwired: 1 in]
                  n572 = Bundle("Axis"=w862, "Histogram"=w861) -> (w863:cluster{"Axis":dbl[], "Histogram":i32[]})  [unwired: 1 in]
                  n573 = property on="ChannelsHist" class="XYGraph (strict)"("Value"=w863) -> ()  [unwired: 2 in, 2 out]
                  n574 = call "crosscorr_sub2.vi"("reference"=w872, "B"="B", "binning"=w871, "macro times 1"=w891, "macro times 2"=w886, "cross ch2 (MCS)"=w857, "cross ch1 (MCS)"=w858, "skip"="skip", "biExp fit"="biExp fit") -> ("crosscorrelation"=w885:cluster{"Tau Values":dbl[], "best fit":dbl[]}[], "F2"=→"F2":dbl, "S+B"=→"S+B (Hz)":dbl, "fit results"=→"results":cluster{dbl, dbl, dbl, dbl, dbl, dbl})  [unwired: 3 in]
                  n575 = local write "Autocorrelation"(w885) -> ()
                }
              }
            }
            frame #3 {
              n576 = local write "Busy"(FALSE ("Busy")) -> ()
            }
          }
        }
        frame #6 {
          n577 = stacked-sequence {
            frame #0 {
              n578 = local write "Busy"(TRUE ("Busy")) -> ()
            }
            frame #1 {
              n579 = stacked-sequence {
                tunnel: "% overtalk D-T1" -> [w915 w931]
                tunnel: "% overtalk D-T2" -> [w916 w930]
                tunnel: "% overtalk D-A" -> [w917 w929]
                frame #0 {
                  n580 = control-ref of="Donor"() -> (w921:refnum<vi>)
                  n581 = control-ref of="Transmitter 1"() -> (w920:refnum<vi>)
                  n582 = property on="HH" class="Boolesch (strikt)"() -> ("Value"=w912:bool)  [unwired: 2 in, 2 out]
                  n583 = control-ref of="Transmitter 2"() -> (w919:refnum<vi>)
                  n584 = control-ref of="bin / s"() -> (w913:refnum<vi>)
                  n585 = control-ref of="Acceptor"() -> (w918:refnum<vi>)
                  n586 = call "F2-alle_sub.vi"("% overtalk D-A"=w917, "% overtalk D-T2"=w916, "% overtalk D-T1"=w915, "binning (s)"=w913, "Channel Akzeptor"=w918, "HydraHarp"=w912, "Channel Transmitter2"=w919, "Channel Transmitter1"=w920, "Channel Donor"=w921) -> ("F2-Values"=→"Fn-Values":cluster{dbl, "Value":dbl, dbl[]}[])
                }
                frame #1 {
                  n587 = local write "# bins"("# bins") -> ()
                  n588 = property on="File Number" class="Slide (strict)"() -> ("Value"=w933:u32)  [unwired: 2 in, 2 out]
                  n589 = property on="channels" class="Array (strict)"() -> ("Value"=w928:u8[])  [unwired: 2 in, 2 out]
                  n590 = control-ref of="# bins"() -> (w943:refnum<vi>)
                  n591 = control-ref of="binning / s"() -> (w942:refnum<vi>)
                  n592 = control-ref of="MCS"() -> (w927:refnum<vi>)
                  n593 = property on="HH" class="Boolesch (strikt)"() -> ("Value"=w922:bool)  [unwired: 2 in, 2 out]
                  n594 = call "Burst7.vi"("# bins"=w943, "binning (s)"=w942, "% overtalk D-T1"=w931, "% overtalk D-T2"=w930, "% overtalk D-A"=w929, "HydraHarp"=w922, "File Number"=w933, "channels"=w928, "x * sigma"="* w0", "MCS"=w927, "Calculate"=TRUE ("overtalk corrrection"), "Parameters"="Parameters", "automatic threshold"="automatic threshold") -> ("mean, std.dev"=→"mean, std.dev":dbl[], "Parameters out"=w924:T34, "Intensity Historgram"=→"Summe":cluster{"Axis":dbl[], "Histogram":i32[]}, "FRET histogram"=w938:cluster{"Axis":dbl[], "Histogram":i32[]}[], "Save F2"=→"Save F2":dbl[][], "Statistik F2"=→"Statistik F2":dbl[], "# bursts"=w941:i32)  [unwired: 8 in]
                  "# bursts" <- w941
                  n595 = property on="Parameters" class="Clust (strict)"("Value"=w924) -> ()  [unwired: 2 in, 2 out]
                  n596 = Greater Or Equal?(x=w941, y=0) -> (x >= y?=w940:bool)
                  n597 = case shown="True" w940 {
                    tunnel: w938 -> [_ w946]
                    frame #0 {
                      n598 = property on="FRET histogram" class="XYGraph (strict)"("Value"=cluster{"Axis":dbl[], "Histogram":i32[]}[] [] ("FRET histogram")) -> ()  [unwired: 2 in, 2 out]
                    }
                    frame #1 {
                      "FRET histogram" <- w946
                    }
                  }
                }
              }
            }
            frame #2 {
              n599 = local write "Busy"(FALSE ("Busy")) -> ()
            }
          }
        }
        frame #7 {
        }
        frame #8 {
          n600 = local read "Tab Control"() -> (w954:T2)
          n601 = call "GetUpdatePanel.vi"("Tab Control"=w954) -> ("Numeric"=w950:u32)
          n602 = Equal?(x=w950, y=u32 8) -> (x = y?=w952:bool)
          n603 = Select(t=i16 4, s=w952, f=w950) -> (s? t:f=w949:u32)
        }
        frame #9 {
          n604 = call "MCS.vi"() -> ("MCS output"=w958:T1)  [unwired: 2 in]
          n605 = Index Array(array=w958, index="channel") -> (element=w956:T18)
          n606 = Unbundle By Name(w956) -> ("Histogram: h(x)"=w955:u32[])
          n607 = stacked-sequence {
            seq-local: [w960 _] -> [_ w985]
            seq-local: [w961 _] -> [_ w984]
            tunnel: w955 -> [w970 _]
            frame #0 {
              n608 = property on="Open" class="Boolesch (strikt)"() -> ("Value"=w965:bool)  [unwired: 2 in, 2 out]
              n609 = case shown="False" w965 {
                tunnel: w970 -> [w978 _]
                tunnel: [w975 w980] -> w962
                tunnel: [w976 w981] -> w963
                frame #0 {
                  n610 = property on="MCS" class="WFGraph (strict)"() -> ("CrsrList"=w974:T15)  [unwired: 2 in, 2 out]
                  n611 = property on="binning / s" class="Digital (strikt)"() -> ("Value"=w977:dbl)  [unwired: 2 in, 2 out]
                  n612 = Index Array(array=w974, index=2) -> (element=w972:T17)
                  n613 = Unbundle By Name(w972) -> ("Position.Y"=w971:dbl)
                  n614 = call "onCounts.vi"("Value"=w971, "Histogram: h(x)"=w978, "binning(s)"=w977) -> ("off times (s)"=w975:dbl[], "on counts"=w976:i32[])
                }
                frame #1 {
                  n615 = property on="off times (s)" class="Array (strikt)"() -> ("Value"=w980:dbl[])  [unwired: 2 in, 2 out]
                  n616 = property on="on counts" class="Array (strikt)"() -> ("Value"=w981:i32[])  [unwired: 2 in, 2 out]
                  n617 = property on="Open" class="Boolesch (strikt)"("Value"=FALSE ("Open")) -> ()  [unwired: 2 in, 2 out]
                }
              }
              n618 = call "previousHist.vi"("in"=w963, "add prev"="add previous") -> ("out"=w961:i32[])
              "on counts" <- w961
              n619 = call "previousOff.vi"("add prev"="add previous", "in"=w962) -> ("out"=w960:dbl[])
              "off times (s)" <- w960
              n620 = call "Std Deviation and Variance.vi"("X"=w960) -> ("mean"=→"off time (s)":dbl, "standard deviation"=→"StdDev":dbl)  [unwired: 1 in, 1 out]
              n621 = call "Std Deviation and Variance.vi"("X"=w961) -> ("mean"=→"on time photons":dbl, "standard deviation"=→"StdDev":dbl)  [unwired: 1 in, 1 out]
            }
            frame #1 {
              n622 = Array Size(array=w984) -> (size(s)=→"# on times":i32)
              n623 = Array Size(array=w985) -> (size(s)=→"# off times":i32)
              n624 = call <vilib>:"Histogram.vi"("intervals"="intervals", "X"=w984) -> ("X Values"=w988:dbl[], "Histogram: h(x)"=w987:i32[])  [unwired: 6 in, 2 out]
              n625 = call <vilib>:"Histogram.vi"("intervals"="intervals", "X"=w985) -> ("X Values"=w991:dbl[], "Histogram: h(x)"=w990:i32[])  [unwired: 6 in, 2 out]
              n626 = Bundle("X Values"=w991, "Histogram: h(x)"=w990) -> (→"off time histogram":T8)  [unwired: 1 in]
              n627 = Bundle("X Values"=w988, "Histogram: h(x)"=w987) -> (→"on count histogram":T8)  [unwired: 1 in]
            }
          }
        }
        frame #10 {
          # "histogram and \ntwo gaussian fit"
          # "E=Acceptor/(Donor+Acceptor)\nin selected range"
          n628 = local read "MCS"() -> (w1021:T1)
          n629 = Unbundle By Name(w1013) -> ("x0"=w1004:dbl, "x1"=w1003:dbl)
          n630 = Index Array(array=w1021, index=1) -> (element=w1018:T18)
          n631 = Index Array(array=w1021, index=4) -> (element=w1017:T18)
          n632 = Unbundle By Name(w1017) -> ("Histogram: h(x)"=w1009:u32[])
          n633 = Unbundle By Name(w1018) -> ("binning (s)"=w1005:dbl, "Histogram: h(x)"=w1012:u32[])
          n634 = Divide(x=w1003, y=w1005) -> (x/y=w1006:dbl)
          n635 = Divide(x=w1004, y=w1005) -> (x/y=w1007:dbl)
          n636 = Subtract(x=w1006, y=w1007) -> (x-y=w1008:dbl)
          n637 = Array Subset(array=w1009, index=w1007, length=w1008) -> (w1010:u32[])
          n638 = Array Subset(array=w1012, index=w1007, length=w1008) -> (w1011:u32[])
          n639 = Add(x=w1011, y=w1010) -> (x+y=w1016:u32[])
          n640 = Divide(x=w1010, y=w1016) -> (x/y=w1015:dbl[])
          n641 = call <vilib>:"General Histogram.vi"("X"=w1015) -> ("Histogram"=w1002:i32[], "Axis"=w998:dbl[])  [unwired: 10 in, 3 out]
          n642 = Bundle("Axis"=w998, "Histogram"=w1002) -> (w1001:cluster{"Axis":dbl[], "Histogram":i32[]})  [unwired: 1 in]
          n643 = case shown="False" "fitting?" {
            tunnel: w1002 -> [_ w1042]
            tunnel: [cluster{"X":dbl[], dbl[]} {"X"=[], []} ("Sum") w1041] -> w999
            tunnel: w998 -> [_ w1040]
            tunnel: [cluster{dbl, dbl, dbl} {0.0, 0.0, 0.0} w1033] -> w995
            frame #0 {
            }
            frame #1 {
              n644 = call "2GaussianFit.vi"("x"=w1040, "Histogram(x)"=w1042) -> ("Sum"=w1041:cluster{"X":dbl[], dbl[]}, "Peak 2"=w1038:dbl[][], "Peak 1"=w1039:dbl[][])
              n645 = Index Array(array=w1038, index (row)=1) -> (element=w1034:dbl[])  [unwired: 1 in]
              n646 = Index Array(array=w1039, index (row)=1) -> (element=w1035:dbl[])  [unwired: 1 in]
              n647 = Add Array Elements(numeric array=w1034) -> (sum=w1025:dbl)
              n648 = Array Max & Min(array=w1034) -> (max index (indices)=w1031:i32)  [unwired: 3 out]
              n649 = Add Array Elements(numeric array=w1035) -> (sum=w1024:dbl)
              n650 = Array Max & Min(array=w1035) -> (max index (indices)=w1032:i32)  [unwired: 3 out]
              n651 = Greater?(x=w1032, y=w1031) -> (0:w1030:bool)
              n652 = Divide(x=w1024, y=w1025) -> (x/y=w1029:dbl)
              n653 = Reciprocal(x=w1029) -> (1/x=w1026:dbl)
              n654 = Bundle(w1024, w1025, w1029) -> (w1028:cluster{dbl, dbl, dbl})  [unwired: 1 in]
              n655 = Bundle(w1025, w1024, w1026) -> (w1027:cluster{dbl, dbl, dbl})  [unwired: 1 in]
              n656 = Select(t=w1028, s=w1030, f=w1027) -> (s? t:f=w1033:cluster{dbl, dbl, dbl})
            }
          }
          n657 = Build Array(w1001, w999) -> (→"Histogram Graph":cluster{"X":dbl[], "Histogram":dbl[]}[])
          n658 = Unbundle(w995) -> (→"area high FRET":dbl, →"area low FRET":dbl, →"ratio peak areas\nFRET high/FRET low":dbl)
          n659 = local write "areas and ratio"(w995) -> ()
        }
      }
      n660 = Not Equal To 0?(x=w391) -> (x != 0?=w394:bool)
    }
  }
